vi "WS1050 36 DUT Reliability HD_Cycling Ver1.3.vi"() -> ()   [LabVIEW 2012]
uses:
  WS_VCAP Driver 029/Source/WSVCAP Shell/Type Defs/WSVCAP SHL I2C DUT Mask Mode Enum.ctl
  <vilib>/Utility/file.llb/Read From Spreadsheet File (DBL).vi
  All Driver/Keithley/2012_Keithley 24XX/Keithley 24XX.lvlib
panel:
  out "VISA resource name out":refnum<visa-resource-name>="GPIB0::3::INSTR"
  out "error out 2":errorcluster={"status"=TRUE, "code"=-63192, "source"="niLvFpga_Open_PXI-7813R.vi"}
  in  "Reg1_Bit Cntrl":string[](array[string])=["01", "02", "04", "08", "10", "20", "40", "80", "03", "06", "0C", "D8", "33", "66", "CC", "07", "0E", "1C", "38", "70", "E0", "0F", "1E", "3C", "78", "F0", "1F", "3E", "7C", "F8", "3F", "7E", "FC", "7F", "FE", "FD", "FB", "F7", "EF", "DF", "BF", "7F", "FC", "F9", "F3", "E7", "CF", "9F", "3F", "F8", "F1", "E3", "C7", "8F", "1F", "F0", "E1", "C3", "87", "0F", "E0", "C1", "83", "07", "C0", "81", "03", "AA", "55", "00"]
  out "date string":string="5/19/2014"
  out "PS1 Out":refnum<visa-resource-name>
  out "Ke2000 Out":refnum<visa-resource-name>="GPIB0::9::INSTR"
  in  "VPI_Cmd":string[](array[string])=["00", "3B", "00"]
  in  "VPI Name":string[](array[string])=["All_Drivers OFF", "All Drivers ON", "All Drivers OFF2"]
  in  "Tab Control":T1(tab)
  in  "No of Cmd":i64=3
  in  "Board#":string="BRD5"
  in  "Serial Number":string[][](table)=[["DUT", "SN"], ["DUT1", "1"], ["DUT2", "2"], ["DUT3", "3"], ["DUT4", "4"], ["DUT5", "5"], ["DUT6", "6"], ["DUT7", "7"], ["DUT8", "8"], ["DUT9", "9"], ["DUT10", "10"], ["DUT11", "11"], ["DUT12", "12"], ["DUT13", "13"], ["DUT14", "14"], ["DUT15", "15"], ["DUT16", "16"], ["DUT17", "17"], ["DUT18", "18"], ["DUT19", "19"], ["DUT20", "20"], ["DUT21", "21"], ["DUT22", "22"], ["DUT23", "23"], ["DUT24", "24"], ["DUT25", "25"], ["DUT26", "26"], ["DUT27", "27"], ["DUT28", "28"], ["DUT29", "29"], ["DUT30", "30"], ["DUT31", "31"], ["DUT32", "32"], ["DUT33", "33"], ["DUT34", "34"], ["DUT35", "35"], ["DUT36", "36"]]
  in  "SPI Clock Rate (Hz)":dbl=5000000.0 caption="Cycle Speed" format="%.1p Hz"
  in  "Wafer#":string="T7-EB"
  in  "File Name":string="CYC_WS1050_T7_EB_65C_40V_25DC_EMPTY_BRD5_141017_1"
  in  "TMN DC\\CAP Data Log File Path":path=path "C:/WS1050 36 DUT Data"
  in  "Test Program":string="WS1050 36 DUT Reliability HD_Cycling Ver1.3"
  out "Current Date":string="8/28/2014"
  out "Current Time":string="0950"
  in  "Start Date":string="10/21/2014"
  in  "Start Time":string="1542"
  in  "Comment":string="CYC65C40V"
  in  "OK Button":bool
  in  "Calibration":bool
  in  "Verify CP":bool
  in  "CP Setting":i32(ring) items=["CP OFF", "CP ON", "CP 35V", "CP 40V", "DVA ON", "DVA OFF", "REG1 ON", "REG1 OFF", "REG2 ON", "REG2 OFF", "REG3 ON", "REG3 OFF"]
  in  "Stop Calibration":bool
  in  "Set VDD":dbl=3.3 format="%.3g"
  in  "Command":string[](array[string])=["07020100003B", "070201003B00", "0702013B0000"]
  in  "Clock Rate (Hz)":dbl=1000000.0 caption="Meas Speed" format="%.1p Hz"
  out "AR  Measurent(Hz)":dbl
  in  "PS1 Source":refnum<visa-resource-name>="GPIB0::5::INSTR"
  in  "Ke2000":refnum<visa-resource-name>="GPIB0::9::INSTR"
  in  "CP to HD/Cycle":i32(ring)=1 items=["CP HDC 35V", "CP HDC 40.25V", "CP HDC 27.5V", "CP HDC 30.5V", "CP HDC 44V"]
  out "Simulate FPGA":bool
  out "Online":bool
  out "AR Cycling(Hz)":dbl=5000000.0
  in  "Ke2400":refnum<visa-resource-name>="GPIB0::3::INSTR"
  in  "Initialize AD7747":bool
  in  "DUT Mask Mode":T2=enum."All"
  in  "RFFE Slave Address":u8=7 caption="Slave Address" format="0x%02x"
  out "Activity Log":string="05/19/2014 -- 12:24:35.853::WSVCAP::APP::Application Started\n05/19/2014 -- 12:24:37.606::WSVCAP::WSVCAP SHL::WR I2C-REG:0x0A;MASK:0xFFFFFFFFFFFF;C1 DATA:22:22:22:22:22:22:22:22:22:22:22:22:22:22:22:22;C2 DATA:22:22:22:22:22:22:22:22:22:22:22:22:22:22:22:22;C3 DATA:22:22:22:22:22:22:22:22:22:22:22:22:22:22:22:22\r\n05/19/2014 -- 12:24:37.773::WSVCAP::WSVCAP SHL::WR I2C-ST:0,0,4,1\r\n05/19/2014 -- 12:24:37.903::WSVCAP::WSVCAP SHL::RD I2C-BYTES:4;ADD:0x00;MASK:0xFFFFFFFFFFFF\r\n05/19/2014 -- 12:24:38.045::WSVCAP::WSVCAP SHL::RD I2C:C1 DATA:2:2:2:2:2:2:2:2:2:2:2:2:2:2:2:2|A7:A9:AA:82:82:7F:82:81:82:81:83:82:81:82:82:81|46:36:BB:88:44:A3:E9:2B:32:20:ED:25:BB:3D:68:B|2C:6A:EB:A7:22:56:FE:CC:36:82:D7:B0:3B:48:F9:CC;C2 DATA:2:2:2:2:2:2:2:2:2:2:2:2:2:2:2:2|94:94:94:80:80:80:80:80:81:7E:7E:81:80:7E:80:80|47:33:15:82:62:B:E8:1C:D7:C3:7D:41:7C:B7:4C:2A|C4:B4:AE:8:1E:D1:4E:37:11:C0:6F:63:42:9D:63:B5;C3 DATA:2:2:2:2:2:2:2:2:2:2:2:2:2:2:2:2|95:95:95:81:81:7E:81:80:84:7D:80:83:81:7E:7F:80|AB:C4:14:B5:7B:52:DF:C9:79:5D:5F:30:99:31:1E:F4|6E:5C:F7:A8:C3:EB:7B:EF:33:92:89:77:4D:67:75:DD;STATUS:0:0:4:0\r\n05/19/2014 -- 12:24:38.046::WSVCAP::WSVCAP SHL::WR I2C-REG:0x0A;MASK:0xFFFFFFFFFFFF;C1 DATA:22:22:22:22:22:22:22:22:22:22:22:22:22:22:22:22;C2 DATA:22:22:22:22:22:22:22:22:22:22:22:22:22:22:22:22;C3 DATA:22:22:22:22:22:22:22:22:22:22:22:22:22:22:22:22\r\n05/19/2014 -- 12:24:38.089::WSVCAP::WSVCAP SHL::WR I2C-ST:0,0,4,1\r\n05/19/2014 -- 12:24:38.219::WSVCAP::WSVCAP SHL::RD I2C-BYTES:4;ADD:0x00;MASK:0xFFFFFFFFFFFF\r\n05/19/2014 -- 12:24:38.362::WSVCAP::WSVCAP SHL::RD I2C:C1 DATA:2:2:2:2:2:2:2:2:2:2:2:2:2:2:2:2|A7:AB:AA:82:82:82:83:83:82:82:82:82:7F:82:82:81|4B:32:96:83:3E:61:43:17:25:62:AB:4D:A2:40:2E:5|3C:76:2B:B4:EE:E4:A9:1A:AA:A:26:C7:21:2E:87:5B;C2 DATA:2:2:2:2:2:2:2:2:2:2:2:2:2:2:2:2|94:94:94:80:80:80:80:80:80:7F:80:81:80:80:7F:80|4A:32:19:7D:19:6C:79:46:61:7F:4B:B8:A5:30:F3:14|B4:70:A:8C:9C:DC:43:FA:1E:A:C6:21:A:A9:13:F3;C3 DATA:2:2:2:2:2:2:2:2:2:2:2:2:2:2:2:2|95:97:94:81:80:81:82:81:80:7E:81:84:7F:81:80:80|B2:32:D0:A7:9E:4C:AB:D4:EE:D9:F0:82:B7:91:7:FF|C1:91:B6:3D:D8:E:1B:4F:9F:6A:F1:6C:E7:3F:7:BA;STATUS:0:0:4:0\r\n05/19/2014 -- 12:24:38.364::WSVCAP::WSVCAP SHL::WR I2C-REG:0x0A;MASK:0xFFFFFFFFFFFF;C1 DATA:22:22:22:22:22:22:22:22:22:22:22:22:22:22:22:22;C2 DATA:22:22:22:22:22:22:22:22:22:22:22:22:22:22:22:22;C3 DATA:22:22:22:22:22:22:22:22:22:22:22:22:22:22:22:22\r\n05/19/2014 -- 12:24:38.406::WSVCAP::WSVCAP SHL::WR I2C-ST:0,0,4,1\r\n05/19/2014 -- 12:24:38.536::WSVCAP::WSVCAP SHL::RD I2C-BYTES:4;ADD:0x00;MASK:0xFFFFFFFFFFFF\r\n05/19/2014 -- 12:24:38.678::WSVCAP::WSVCAP SHL::RD I2C:C1 DATA:2:2:2:2:2:2:2:2:2:2:2:2:2:2:2:2|A7:A9:AB:82:82:81:82:82:82:82:82:82:82:82:82:81|46:71:4C:87:43:3D:7F:FC:25:4F:8E:54:97:3E:60:8C|AA:F4:1F:B5:CE:43:1F:36:9:87:9C:78:86:5:B6:8E;C2 DATA:2:2:2:2:2:2:2:2:2:2:2:2:2:2:2:2|94:94:94:80:7F:7F:80:80:80:80:80:81:80:80:80:80|49:36:18:7D:6E:C5:E4:3C:81:2E:41:D3:75:71:E3:72|E8:D3:E6:D1:E0:48:AE:D4:54:D:E8:8E:B4:41:68:4;C3 DATA:2:2:2:2:2:2:2:2:2:2:2:2:2:2:2:2|95:95:95:81:7F:7F:81:81:81:81:81:84:81:81:82:81|B3:F5:90:AB:82:69:7B:93:D0:77:E8:D5:E8:8C:84:E8|B9:AC:EE:2B:B6:71:8F:4A:74:31:56:BB:8A:B7:A0:C8;STATUS:0:0:4:0\r\n05/19/2014 -- 12:24:38.681::WSVCAP::WSVCAP SHL::WR I2C-REG:0x0A;MASK:0xFFFFFFFFFFFF;C1 DATA:22:22:22:22:22:22:22:22:22:22:22:22:22:22:22:22;C2 DATA:22:22:22:22:22:22:22:22:22:22:22:22:22:22:22:22;C3 DATA:22:22:22:22:22:22:22:22:22:22:22:22:22:22:22:22\r\n05/19/2014 -- 12:24:38.723::WSVCAP::WSVCAP SHL::WR I2C-ST:0,0,4,1\r\n05/19/2014 -- 12:24:38.854::WSVCAP::WSVCAP SHL::RD I2C-BYTES:4;ADD:0x00;MASK:0xFFFFFFFFFFFF\r\n05/19/2014 -- 12:24:38.996::WSVCAP::WSVCAP SHL::RD I2C:C1 DATA:2:2:2:2:2:2:2:2:2:2:2:2:2:2:2:2|A7:A9:AA:82:82:7F:83:81:82:81:84:82:7F:82:7F:82|43:FB:E:7F:3C:AD:35:35:26:A2:6C:21:4B:3D:8:6|63:9A:E1:F3:95:32:91:42:90:3C:78:1F:5C:D7:5F:D8;C2 DATA:2:2:2:2:2:2:2:2:2:2:2:2:2:2:2:2|94:94:94:80:80:80:80:80:81:80:7E:81:80:7E:7F:80|48:36:18:7F:5E:3D:69:83:DE:AE:A1:9E:31:AE:BB:96|15:A0:44:17:13:FD:CC:C8:6D:B2:EF:A7:C:C7:3B:F;C3 DATA:2:2:2:2:2:2:2:2:2:2:2:2:2:2:2:2|95:96:94:81:81:7E:82:80:84:80:80:84:7F:7E:7D:82|AD:3B:6D:A9:7C:57:9D:F5:7A:96:23:5C:36:2D:ED:5A|CD:46:DB:3B:C7:BD:70:60:33:B8:B:F7:63:A:51:4D;STATUS:0:0:4:0\r\n05/19/2014 -- 12:24:38.998::WSVCAP::WSVCAP SHL::WR I2C-REG:0x0A;MASK:0xFFFFFFFFFFFF;C1 DATA:22:22:22:22:22:22:22:22:22:22:22:22:22:22:22:22;C2 DATA:22:22:22:22:22:22:22:22:22:22:22:22:22:22:22:22;C3 DATA:22:22:22:22:22:22:22:22:22:22:22:22:22:22:22:22\r\n05/19/2014 -- 12:24:39.040::WSVCAP::WSVCAP SHL::WR I2C-ST:0,0,4,1\r\n05/19/2014 -- 12:24:39.170::WSVCAP::WSVCAP SHL::RD I2C-BYTES:4;ADD:0x00;MASK:0xFFFFFFFFFFFF\r\n05/19/2014 -- 12:24:39.311::WSVCAP::WSVCAP SHL::RD I2C:C1 DATA:2:2:2:2:2:2:2:2:2:2:2:2:2:2:2:2|A7:AA:AB:82:82:81:82:81:82:81:82:82:82:82:7F:82|44:F1:90:87:45:44:C8:2C:2C:F1:FC:1B:94:3B:3C:75|4A:49:95:19:99:73:64:3:23:24:F3:A2:5E:7F:C4:B6;C2 DATA:2:2:2:2:2:2:2:2:2:2:2:2:2:2:2:2|94:94:94:80:80:80:80:7F:80:80:7E:80:80:7E:7F:80|4C:36:17:7D:A8:9F:DE:C7:53:6D:8A:F4:41:A5:C6:E0|90:2E:24:C:D9:22:E4:76:3B:40:1D:53:33:B1:3E:4D;C3 DATA:2:2:2:2:2:2:2:2:2:2:2:2:2:2:2:2|95:97:95:81:81:7F:81:80:80:81:7F:82:81:7E:7D:82|AE:2B:A7:AB:CC:CD:A4:38:FD:17:80:F2:92:2D:45:C4|76:E5:D:B9:AD:B5:BA:8D:28:32:9E:42:B7:20:4A:D9;STATUS:0:0:4:0\r\n05/19/2014 -- 12:24:39.313::WSVCAP::WSVCAP SHL::WR I2C-REG:0x0A;MASK:0xFFFFFFFFFFFF;C1 DATA:22:22:22:22:22:22:22:22:22:22:22:22:22:22:22:22;C2 DATA:22:22:22:22:22:22:22:22:22:22:22:22:22:22:22:22;C3 DATA:22:22:22:22:22:22:22:22:22:22:22:22:22:22:22:22\r\n05/19/2014 -- 12:24:39.355::WSVCAP::WSVCAP SHL::WR I2C-ST:0,0,4,1\r\n05/19/2014 -- 12:24:39.486::WSVCAP::WSVCAP SHL::RD I2C-BYTES:4;ADD:0x00;MASK:0xFFFFFFFFFFFF\r\n05/19/2014 -- 12:24:39.628::WSVCAP::WSVCAP SHL::RD I2C:C1 DATA:2:2:2:2:2:2:2:2:2:2:2:2:2:2:2:2|A7:A9:AA:82:82:82:83:82:82:82:82:82:7F:82:7F:82|47:18:E4:87:3E:E7:6:65:25:92:37:38:A8:3E:89:85|7C:A7:7:2B:A3:7A:EC:EF:89:ED:F4:D3:D8:BC:3A:F5;C2 DATA:2:2:2:2:2:2:2:2:2:2:2:2:2:2:2:2|94:94:94:80:7F:80:80:7F:81:80:7E:80:80:80:81:80|49:37:17:80:76:25:6A:F8:DF:55:97:4D:B8:5B:2B:B1|13:E3:9A:3E:1A:2D:4F:B6:DB:E9:61:FA:8B:D6:9:CC;C3 DATA:2:2:2:2:2:2:2:2:2:2:2:2:2:2:2:2|95:95:95:81:7F:80:82:81:84:80:7F:81:80:81:7F:82|AF:93:3B:AF:5B:11:82:E4:7E:C3:2D:72:9:96:D9:A|DB:96:F2:10:5F:64:9A:C6:98:12:27:7D:10:D3:20:D9;STATUS:0:0:4:0\r\n05/19/2014 -- 12:24:40.132::WSVCAP::WSVCAP SHL::CLOSE\r\n"
  in  "C1 Cap DAC":u8=128 caption="B Data In" format="0x%02x"
  in  "C2 Cap DAC":u8=128 caption="B Data In" format="0x%02x"
  in  "C3 Cap DAC":u8=128 caption="B Data In" format="0x%02x"
  out "IDD Brd(uA)":string
  in  "CP to Meas":i32(ring)=1 items=["CP HDC 35V", "CP HDC 40.25V", "CP HDC 27.5V", "CP HDC 30.5V", "CP HDC 44V"]
  in  "CP VPI":i32(ring) items=["CP HDC 35V", "CP HDC 40.25V", "CP HDC 27.5V", "CP HDC 30.5V", "CP HDC 44V"]
  in  "Repeat Meas(s)":u32=900
  in  "Real No. From\nLookup Table":bool
  in  "Control Panel":T3={"Verify Socket"=FALSE, "HD/CYC"=FALSE, "E-CAL"=FALSE, "DVA"=FALSE, "VPI"=TRUE, "VSA"=TRUE, "HS"=TRUE}
  out "Verify Socket":bool
  out "HD/CYC":bool
  out "E-CAL":bool
  out "DVA":bool
  out "VPI":bool
  out "VSA":bool
  out "HS":bool
  in  "Lot#":string="WS1050"
  out "AD7747 Values":string[][](table)
  in  "Freq(Hz)":string="12K"
  in  "Reset P/S":bool
  in  "Test Sequences":i32(ring) items=["C1_C2_C3", "C2_C1_C3", "C3_C2_C1"]
  in  "WS1050/51":bool=TRUE
  in  "CP with DVA ON":i32(ring) items=["CP HDC 35V", "CP HDC 40.25V", "CP HDC 27.5V", "CP HDC 30.5V", "CP HDC 44V"]
  in  "% Duty Cycle":string="33"
  in  "Cmd To HD":string="0702013B3B3B"
  in  "Post CMd Delay":dbl[](array[numeric])=[1.8e-05, 1.8e-05, 1.8e-05] min=0.0 max=0.5 format="%#.0p s"
  in  "Cmin/Act":bool=TRUE
  out "40V_1":string[][](table)
  out "NOM IDD OFF(uA)":string
  out "40V_2":string[][](table)
  out "40V_3":string[][](table)
  out "Total Time":u64
  in  "Set HD/Cycle \nto Complete":u64=50000000000
  out "No of HD/Cycle\nCompleted":u64
  out "Cycle Count":u64 min=1 max=4 step=1
  out "Loop \ncompleted":i32=1
  out "Previous Time":string="12:20:26 PM"
  out "STATUS":string="Idle...."
  out "Total Delta C2(pF)":string[](array[string])
  out "Total Delta C1(pF)":string[](array[string])
  out "Total Delta C3(pF)":string[](array[string])
  out "RB Reg for HD":string[](array[string])
  out "RB Reg for HD/Cycle":string[](array[string])
  out "VPI C2":string[][](table)
  out "VPI C3":string[][](table)
  out "NOM IDD ON (uA)":string
  out "IDD_HD/CYC (uA)":string="164.601255E+0"
  in  "stop During HD/Cycles":bool
  in  "stop":bool
  out "IDD Stdby(uA)":string="2.606990E+0"
  out "VPI C1":string[][](table)
  out "VSA_V1":string[][](table)
  out "VSA_V2":string[][](table)
  out "VSA_V3":string[][](table)
  in  "VSA Voltage(V)":dbl[](array[numeric])=[-10.0, 0.0, 10.0]
  in  "DC_Temp":i32=65
  in  "HD/CYC Temp":i32=65
  in  "Time All ON (s)":u32=120
  in  "Time All OFF (s)":u32=120
  in  "HD_DC (Min)":u64=259200
  out "LPs Count":i32
  in  "X Repeat":i32=100
  out "No LPs to RP":i32
  out "Run Loops":i32=1
  out "TTCompleted":u64=2000
  in  "TTF Completed":u64=50000000000
  out "% Delta C_T0":string[][](array[string])
  out "% Delta C":string[][](array[string])
  out "EFuse RB T0":string[](array[string])
  out "Current EFuse Read back":string[](array[string])
  out "EFuse Readback Status":bool[](array[boolean])
  in  "DeltaC Target Setting(pF)":dbl=7.375
  out "error out":errorcluster
  in  "error in (no error)":errorcluster
  in  "HD RP":dbl=60.0
  in  "Cycle RP":dbl=10000.0
  out "Min Plot_1":dbl[][](graph) caption="(Y) Multi Plot 2"
  out "Min Plot_2":dbl[][](graph) caption="(Y) Multi Plot 2"
  out "Min Plot_3":dbl[][](graph) caption="(Y) Multi Plot 2"
  in  "Debug":bool
  in  "No of Rows\nFrom Spread Sheet":i32
  in  "Plot Delta Cmin":bool=TRUE
  in  "Plot":T4(ring)
  # "Company:  WiSpry Inc\n20 Fairbanks Ste 198 Irvine CA 92618\n\nAuthor:  Andy V Tran\nCreated:  03/19/2015\nLabVIEW 2012 Pro\nTest Program:  WS1050 36 DUT Reliability HD_Cycling ver1.3\nFPGA: WS_VCAP Driver 029"
  # "Note for HD Duty Cycle:\n1.  Set time to start HD_DC (Min), default is 259200 (6 months) \n2.  Set Time for Duty Cycle ON/OFF, default setting is 2 minutes\n3.  No of Loops to RP = 3600s/(Time ALL ON(s) + Time ALL + OFF(s))\n4.  Set X Repeat = no of runs, default is 100 runs\n5.  Set TTF Completed to stop the test.\n\nVer 1.3 updated:\n1.  Added stress sequences; CMin/ON-OFF repeat measurement\n2.  Fill \"na\" to preadsheet with no test"
  # "Minutes"
  # "X1000"
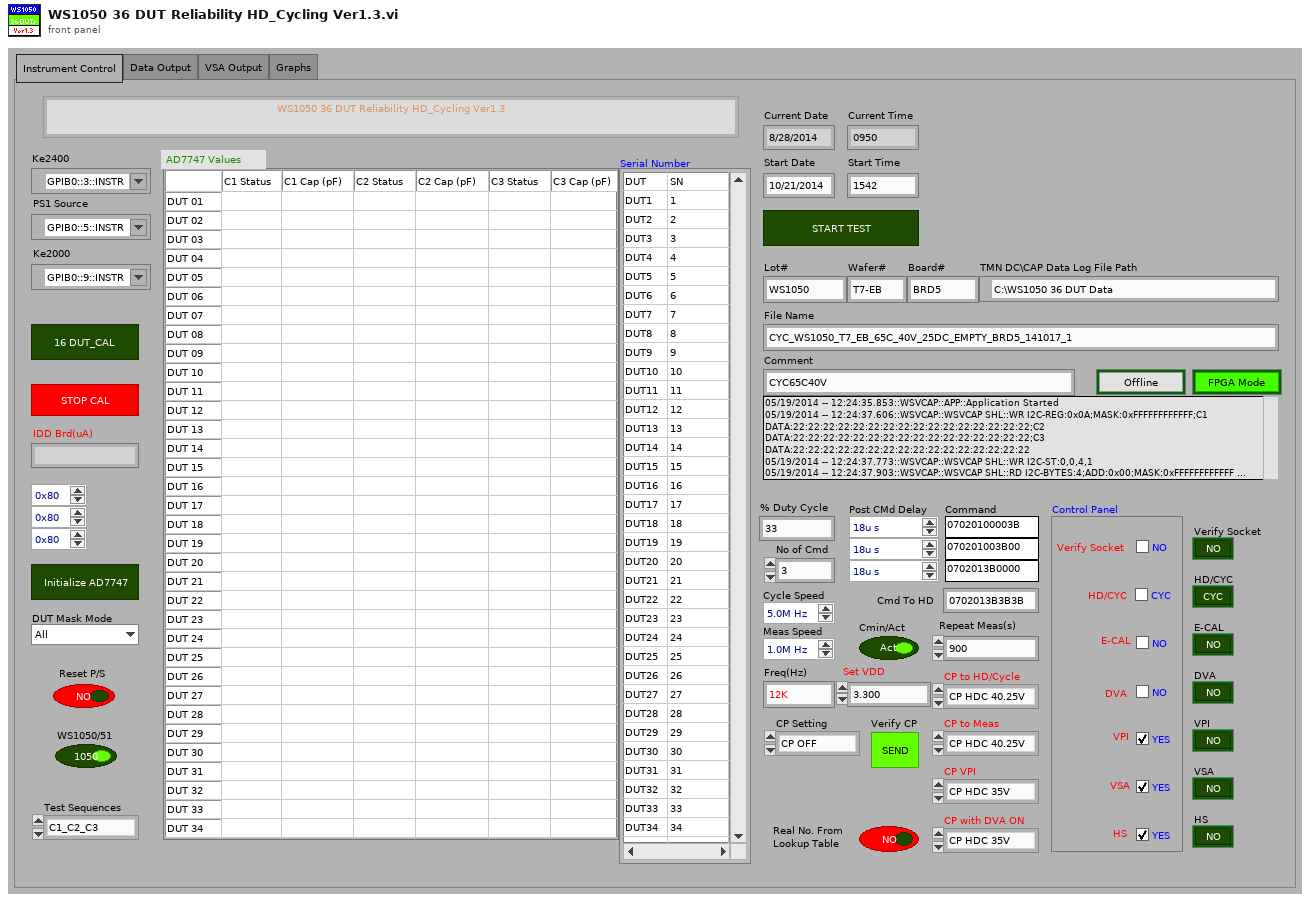
[diagram p1: front panel]
types:
  T1 = enum32{"Instrument Control", "Data Output", "VSA Output", "Graphs"}
  T2 = typedef "WSVCAP SHL I2C DUT Mask Mode Enum.ctl" = enum16{"Custom", "C1", "C2", "C3", "All"}
  T3 = cluster{"Verify Socket":bool, "HD/CYC":bool, "E-CAL":bool, "DVA":bool, "VPI":bool, "VSA":bool, "HS":bool}
  T4 = enum16{"ALL DUTs", "DUT 01", "DUT 02", "DUT 03", "DUT 04", "DUT 05", "DUT 06", "DUT 07", "DUT 08", "DUT 09", "DUT 10", "DUT 11", "DUT 12", "DUT 13", "DUT 14", "DUT 15", "DUT 16", "DUT 17", "DUT 18", "DUT 19", "DUT 20", "DUT 21", "DUT 22", "DUT 23", "DUT 24", "DUT 25", "DUT 26", "DUT 27", "DUT 28", "DUT 29", "DUT 30", "DUT 31", "DUT 32", "DUT 33", "DUT 34", "DUT 35", "DUT 36"}
  T5 = typedef "WSVCAP SHL Core System Cluster.ctl" = cluster{"Settings":T6, "FPGA Resource":tag, "Online":bool, "I2C Wait Ticks":u32, "SPI Wait Ticks":u32, "RFFE Wait Ticks":u32}
  T6 = typedef "WSVCAP SHL I2C Settings Cluster.ctl" = cluster{"FPGA Resource Name":string, "I2C Slave Address":u8, "I2C Clock Rate (Hz)":dbl, "SPI Clock Rate (Hz)":dbl, "RFFE Slave Address":u8, "RFFE Clock Rate (Hz)":dbl, "Simulate FPGA":bool, "C1 Cap DAC Default":u8, "C2 Cap DAC Default":u8, "C3 Cap DAC Default":u8}
  T7 = enum16{"Idle...", "Voltage 1", "Voltage 2", "Voltage 3"}[]
  T8 = cluster{"Test Program ":string, "Comment":string, "Data Out":string, "Data Out":string, "Data Out":string, string, "Data Out":string, "Data Out":string, "string":string, "Freq(Hz)":string, "Board#":string}
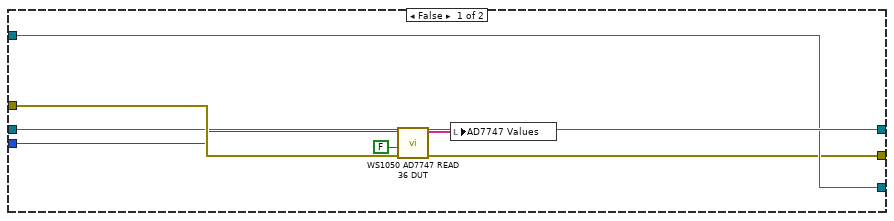
[diagram p10: hidden frame]
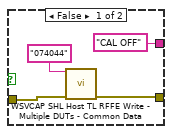
[diagram p11: hidden frame]
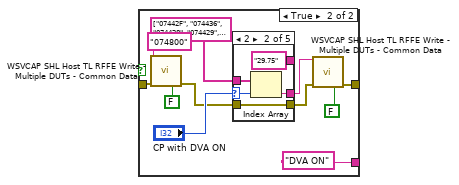
[diagram p12: hidden frame]
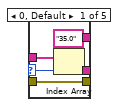
[diagram p13: hidden frame]
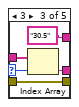
[diagram p14: hidden frame]
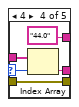
[diagram p15: hidden frame]
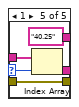
[diagram p16: hidden frame]
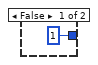
[diagram p17: hidden frame]
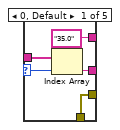
[diagram p18: hidden frame]
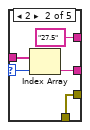
[diagram p19: hidden frame]
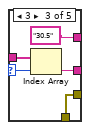
[diagram p20: hidden frame]
diagram:
  w19 = TRUE
  w25 = u16 0 items=["Off", "Moving Filter", "Repeating Filter"] ("Digital Filter (0: Off)")
  w26 = u16 7 items=["3.5 Digits"=4, "4.5 Digits"=5, "5.5 Digits"=6, "6.5 Digits"=7] ("Resolution (7: 6.5 digits)")
  n1 = case shown="True" w19 {
    tunnel: "error in (no error)" -> [w33 w34]
    tunnel: [w33 w41] -> w5
    frame False {
    }
    frame True {
      n2 = call "WSVCAP SHL Host TL Initialize.vi"("error in"=w34) -> ("error out"=w35:errorcluster)  [unwired: 13 in, 1 out]
      n3 = control-ref of="Activity Log"() -> (w37:refnum<vi>)
      n4 = call "ACT LG Activity Log Core.vi"("Display Ref"=w37, "Source"="WSVCAP", "Error In (no error)"=w35) -> ("Error Out"=w36:errorcluster)  [unwired: 11 in, 1 out]
      n5 = call "WSVCAP SHL Host TL Status Manager.vi"("error in"=w36) -> ("System Out"=w42:T5, "error out"=w41:errorcluster)  [unwired: 13 in]
      n6 = Unbundle By Name(w42) -> ("Online"=→"Online":bool, "Settings.Simulate FPGA"=→"Simulate FPGA":bool)
    }
  }
  n7 = case shown="True" TRUE {
    tunnel: w5 -> [w43 w48]
    tunnel: [w44 w47] -> w16
    tunnel: [w43 w46] -> w9
    tunnel: "Ke2400" -> [w44 w45]
    frame False {
    }
    frame True {
      n8 = VISA Write(VISA resource name=w45, write buffer="SOUR:FUNC VOLT;VOLT:MODE FIX;RANG 100;LEV 0.0;:SENS:FUNC \"CURR\";CURR:PROT 60E-3;RANG 100E-3;:OUTP ON", error in (no error)=w48) -> (VISA resource name out=w47:refnum<visa-resource-name>, error out=w46:errorcluster)  [unwired: 1 out]
    }
  }
  n9 = case shown="True" "Reset P/S" {
    tunnel: "PS1 Source" -> [w50 w57]
    tunnel: [w50 w55] -> w30
    tunnel: w5 -> [w51 w53]
    tunnel: [w51 w52] -> w4
    frame False {
    }
    frame True {
      n10 = call "Agilent 3631A Initialize.vi"("error in (no error)"=w53, "Default"=FALSE ("Reset? (T: Yes)"), "Reset"=TRUE ("ID Query? (T: Yes)"), "VISA resource name"=w57) -> ("error out"=w52:errorcluster, "VISA resource name out"=w55:refnum<visa-resource-name>)  [unwired: 6 in]
    }
  }
  n11 = call "Ke2000 Initialize.vi"("error in (no error)"=w5, "VISA resource name"="Ke2000") -> ("error out"=w27:errorcluster, "VISA resource name out"=w28:refnum<visa-resource-name>)  [unwired: 8 in]
  n12 = call "Ke2000 Configure DC Current.vi"("Resolution (7: 6.5 digits)"=w26, "Digital Filter (0: Off)"=w25, "Auto Range? (T: Auto)"=FALSE, "error in (no error)"=w27, "Custom Range (0 A)"=1.0, "VISA resource name"=w28) -> ("error out"=w6:errorcluster, "VISA resource name out"=w23:refnum<visa-resource-name>)  [unwired: 4 in]
  n13 = case shown="True" TRUE {
    tunnel: [_ w58] -> w32
    frame False {
    }
    frame True {
      n14 = call-poly <vilib>:"Read From Spreadsheet File.vi"("number of rows (all:-1)"=-1) -> ("all rows"=w58:dbl[][])  [unwired: 6 in, 4 out]
    }
  }
  n15 = Merge Errors(w9, w6, w4) -> (w17:errorcluster)
  n16 = while {
    tunnel: w17 -> [w62]
    tunnel: [w71] -> w13
    tunnel: w32 -> [w87]
    tunnel: w30 -> [w75]
    tunnel: w23 -> [w76]
    tunnel: [w85] -> w22
    tunnel: [w84] -> w21
    tunnel: w16 -> [w82]
    tunnel: [w81] -> w14
    tunnel: [FALSE ("stop")] -> w7
    i -> [w83]
    stop <- w88 stop-if-true
    n17 = case shown="0" w83 {
      tunnel: w62 -> [w99 w101]
      tunnel: [w98 w101] -> w78
      tunnel: "RFFE Slave Address" -> [w96 _]
      frame 0 {
        w92 = dbl[][] []
        w91 = "" ("uA")
        w93 = string[][] []
        w94 = string[] [] ("EFuse Read back")
        w100 = u64 0 ("No of HD/Cycle\nCompleted")
        n18 = local write "RB Reg for HD/Cycle"(w94) -> ()
        n19 = local write "Current EFuse Read back"(w94) -> ()
        n20 = local write "EFuse RB T0"(w94) -> ()
        n21 = local write "Total Delta C1(pF)"(w94) -> ()
        n22 = local write "Total Delta C2(pF)"(w94) -> ()
        n23 = local write "Total Delta C3(pF)"(w94) -> ()
        n24 = local write "No of HD/Cycle\nCompleted"(w100) -> ()
        n25 = local write "Cycle Count"(w100) -> ()
        n26 = local write "VPI C2"(w93) -> ()
        n27 = local write "VSA_V3"(w93) -> ()
        n28 = local write "VSA_V1"(w93) -> ()
        n29 = local write "40V_2"(w93) -> ()
        n30 = local write "40V_1"(w93) -> ()
        n31 = local write "NOM IDD OFF(uA)"(w91) -> ()
        n32 = local write "NOM IDD ON (uA)"(w91) -> ()
        n33 = local write "IDD Brd(uA)"(w91) -> ()
        n34 = local write "VSA_V2"(w93) -> ()
        n35 = local write "VPI C1"(w93) -> ()
        n36 = local write "VPI C3"(w93) -> ()
        n37 = local write "% Delta C"(w93) -> ()
        n38 = local write "% Delta C_T0"(w93) -> ()
        n39 = local write "40V_3"(w93) -> ()
        n40 = call "WSVCAP SHL Host TL RFFE Configure.vi"("RFFE Slave Address"=w96, "Clock Rate (Hz)"="Clock Rate (Hz)", "error in"=w99) -> ("Actual Rate (Hz)"=→"AR  Measurent(Hz)":dbl, "error out"=w98:errorcluster)  [unwired: 11 in]
        n41 = local write "Min Plot_3"(w92) -> ()
        n42 = local write "Min Plot_1"(w92) -> ()
        n43 = local write "Min Plot_2"(w92) -> ()
      }
      frame 1, Default {
      }
    }
    n44 = while {
      tunnel: ["stop"] -> w80
      tunnel: w78 -> [w127]
      tunnel: [w119] -> w72
      tunnel: w75 -> [w126]
      tunnel: w76 -> [w121]
      tunnel: [w122] -> w74
      tunnel: [w120] -> w73
      tunnel: [w117] -> w69
      tunnel: [w116] -> w68
      tunnel: [w115] -> w67
      tunnel: [w114] -> w66
      tunnel: [w113] -> w65
      tunnel: [w112] -> w64
      tunnel: [w111] -> w63
      tunnel: ["Command"] -> w61
      tunnel: ["Post CMd Delay"] -> w60
      stop <- w134 stop-if-true
      # "Set Date & Time to Start Test"
      n45 = case shown="True" "Initialize AD7747" {
        tunnel: w127 -> [w143 w148]
        tunnel: [w143 w144] -> w110
        tunnel: w126 -> [w142 w146]
        tunnel: [w142 w145] -> w125
        frame False {
        }
        frame True {
          w149 = T7 [enum."Voltage 2", enum."Voltage 3", enum."Voltage 1"] items=["Idle...", "Voltage 1", "Voltage 2", "Voltage 3"]
          n46 = for {
            tunnel: w146 -> [w159]
            tunnel: w149 -> [w157] mode=indexing
            tunnel: [w156] -> w145
            shift-right: [w152] -> w147
            shift-left: w148 -> [w160]
            n47 = local read "Set VDD"() -> (w155:dbl)
            n48 = call "E3631A_Voltage Controller.vi"("VISA resource name"=w159, "I_VDD(A)"=0.5, "Channel Controller"=w157, "Voltage 1"=w155, "Voltage 2"=3.3, "error in (no error)"=w160, "I_3.3V (A)"=0.5) -> ("VISA resource name out"=w156:refnum<visa-resource-name>, "error out"=w151:errorcluster)  [unwired: 7 in]
            n49 = call "Delay T4.vi"("milliseconds to wait"=u32 100, "error in (no error)"=w151) -> ("error out"=w152:errorcluster)  [unwired: 9 in]
          }
          n50 = call "WS1050_AD7747_Init 36DUT.vi"("error in"=w147) -> ("error out"=w144:errorcluster)  [unwired: 10 in]
        }
      }
      n51 = call "Time_stamp.vi"() -> ("date/time string"=w139:string, "date string"=w141:string)  [unwired: 2 in]
      "Current Date" <- w141
      "Current Time" <- w139
      n52 = Equal?(x=w141, y="Start Date") -> (x = y?=w137:bool)
      n53 = Equal?(x=w139, y="Start Time") -> (x = y?=w136:bool)
      n54 = And(x=w137, y=w136) -> (x .and. y?=w133:bool)
      n55 = Compound Arithmetic op=OR(w133, "OK Button", "stop") -> (w134:bool)
      n56 = case shown="True" "Calibration" {
        tunnel: w110 -> [w190 w207]
        tunnel: [w184 w204] -> w108
        tunnel: w125 -> [w189 w203]
        tunnel: "DUT Mask Mode" -> [w188 w199]
        tunnel: [w189 w198] -> w123
        tunnel: w121 -> [w187 w194]
        tunnel: [w187 w191] -> w120
        frame False {
          n57 = call "WS1050 AD7747 READ 36 DUT.vi"("error in"=w190, "Log (T)"=FALSE, "DUT Mask Mode (All)"=w188) -> ("error out"=w184:errorcluster, "AD7747 Values"=w185:string[][])  [unwired: 7 in]
          n58 = local write "AD7747 Values"(w185) -> ()
        }
        frame True {
          n59 = flat-sequence {
            tunnel: w207 -> [w216]
            tunnel: [w211] -> w206
            tunnel: w203 -> [w215]
            tunnel: [w214] -> w202
            tunnel: w199 -> [w213]
            tunnel: [w213] -> w200
            tunnel: w194 -> [w209]
            tunnel: [w208] -> w193
            tunnel: w206 -> [w240]
            tunnel: [w239] -> w205
            tunnel: w202 -> [w238]
            tunnel: [w238] -> w201
            tunnel: w200 -> [w237]
            tunnel: "C1 Cap DAC" -> [w233]
            tunnel: "C2 Cap DAC" -> [w232]
            tunnel: "C3 Cap DAC" -> [w231]
            tunnel: w193 -> [w230]
            tunnel: [w230] -> w192
            tunnel: w205 -> [w249]
            tunnel: [w252] -> w204
            tunnel: w201 -> [w251]
            tunnel: [w248] -> w198
            tunnel: w192 -> [w247]
            tunnel: [w247] -> w191
            frame #0 {
              w217 = T7 [enum."Voltage 2", enum."Voltage 3", enum."Voltage 1"] items=["Idle...", "Voltage 1", "Voltage 2", "Voltage 3"]
              n60 = for {
                tunnel: w215 -> [w228]
                tunnel: w217 -> [w226] mode=indexing
                tunnel: [w225] -> w214
                shift-right: [w223] -> w210
                shift-left: w216 -> [w229]
                n61 = local read "Set VDD"() -> (w220:dbl)
                n62 = call "E3631A_Voltage Controller.vi"("VISA resource name"=w228, "I_VDD(A)"=0.5, "Channel Controller"=w226, "Voltage 1"=w220, "Voltage 2"=3.3, "error in (no error)"=w229, "I_3.3V (A)"=0.5) -> ("VISA resource name out"=w225:refnum<visa-resource-name>, "error out"=w222:errorcluster)  [unwired: 7 in]
                n63 = call "Delay T4.vi"("milliseconds to wait"=u32 100, "error in (no error)"=w222) -> ("error out"=w223:errorcluster)  [unwired: 9 in]
              }
              n64 = call "Ke2000 Single Reading.vi"("error in (no error)"=w210, "VISA resource name"=w209) -> ("error out"=w211:errorcluster, "VISA resource name out"=w208:refnum<visa-resource-name>, "uA"=→"IDD Brd(uA)":string)  [unwired: 5 in, 2 out]
              n65 = One Button Dialog(message="Please verify all sockets should be empty...") -> ()  [unwired: 1 in, 1 out]
            }
            frame #1 {
              n66 = call "WS1050 CAPDAC Setting.vi"("DUT Mask Mode (All)"=w237, "error in"=w240, "C3 Cap DAC"=w231, "C2 Cap DAC"=w232, "C1 Cap DAC"=w233) -> ("error out"=w235:errorcluster)  [unwired: 5 in, 1 out]
              n67 = call "WS1050 OFFSET CAL.vi"("error in"=w235, "OFFSET CAL"=TRUE ("Read?")) -> ("error out"=w234:errorcluster)  [unwired: 8 in, 1 out]
              n68 = while {
                tunnel: w234 -> [w246]
                tunnel: [w245] -> w239
                tunnel: w237 -> [w243]
                stop <- "Stop Calibration" stop-if-true
                n69 = call "WS1050 AD7747 READ 36 DUT.vi"("error in"=w246, "Log (T)"=FALSE, "DUT Mask Mode (All)"=w243) -> ("error out"=w245:errorcluster, "AD7747 Values"=→"AD7747 Values":string[][])  [unwired: 7 in]
              }
            }
            frame #2 {
              w250 = T7 [enum."Voltage 2", enum."Voltage 3", enum."Voltage 1"] items=["Idle...", "Voltage 1", "Voltage 2", "Voltage 3"]
              n70 = for {
                tunnel: w251 -> [w264]
                tunnel: w250 -> [w261] mode=indexing
                tunnel: [w260] -> w248
                shift-right: [w256] -> w252
                shift-left: w249 -> [w262]
                n71 = call "E3631A_Voltage Controller.vi"("VISA resource name"=w264, "I_VDD(A)"=0.5, "Channel Controller"=w261, "Voltage 1"=0.0, "Voltage 2"=3.3, "error in (no error)"=w262, "I_3.3V (A)"=0.5) -> ("VISA resource name out"=w260:refnum<visa-resource-name>, "error out"=w255:errorcluster)  [unwired: 7 in]
                n72 = call "Delay T4.vi"("milliseconds to wait"=u32 100, "error in (no error)"=w255) -> ("error out"=w256:errorcluster)  [unwired: 9 in]
              }
              n73 = One Button Dialog(message="Calibration Completed....") -> ()  [unwired: 1 in, 1 out]
            }
          }
        }
      }
      n74 = call "Control Panel.vi"("error in (no error)"=w110, "Control Panel"="Control Panel") -> ("error out"=w107:errorcluster, "VPI"=w113:bool, "DVA"=w114:bool, "E-CAL"=w115:bool, "VSA"=w112:bool, "HD/CYC"=w116:bool, "HS"=w111:bool, "Verify Socket"=w117:bool)  [unwired: 2 in]
      "Verify Socket" <- w117
      "E-CAL" <- w115
      "VPI" <- w113
      "VSA" <- w112
      "HS" <- w111
      "HD/CYC" <- w116
      "DVA" <- w114
      n75 = Merge Errors(w107, w108) -> (w109:errorcluster)
      n76 = case shown="True" "Verify CP" {
        tunnel: [w161 w165] -> w119
        tunnel: w123 -> [w162 w168]
        tunnel: [w162 w166] -> w122
        tunnel: w109 -> [w161 w164]
        frame False {
        }
        frame True {
          w169 = T7 [enum."Voltage 2", enum."Voltage 3", enum."Voltage 1"] items=["Idle...", "Voltage 1", "Voltage 2", "Voltage 3"]
          # "Verify CP"
          n77 = for {
            tunnel: w168 -> [w182]
            tunnel: w169 -> [w180] mode=indexing
            shift-right: [w177] -> w167
            shift-left: w164 -> [w183]
            tunnel: [w175] -> w166
            n78 = local read "Set VDD"() -> (w179:dbl)
            n79 = call "E3631A_Voltage Controller.vi"("VISA resource name"=w182, "I_VDD(A)"=0.5, "Channel Controller"=w180, "Voltage 1"=w179, "Voltage 2"=3.3, "error in (no error)"=w183, "I_3.3V (A)"=0.5) -> ("VISA resource name out"=w175:refnum<visa-resource-name>, "error out"=w178:errorcluster)  [unwired: 7 in]
            n80 = call "Delay T4.vi"("milliseconds to wait"=u32 100, "error in (no error)"=w178) -> ("error out"=w177:errorcluster)  [unwired: 9 in]
          }
          n81 = Index Array(array=string[] ["074000", "074040", "07476F", "074776", "074800", "074820", "07413B", "074100", "07423B", "074200", "07433B", "074300"], index="CP Setting") -> (element=w170:string)
          n82 = call "WSVCAP SHL Host TL RFFE Write - Multiple DUTs - Common Data.vi"("Data Out"=w170, "error in"=w167, "Log (T)"=FALSE) -> ("error out"=w165:errorcluster)  [unwired: 12 in]
        }
      }
      n83 = Array Subset(array="Post CMd Delay", length="No of Cmd") -> (w105:dbl[])  [unwired: 1 in]
      n84 = Array Subset(array="Command", length="No of Cmd") -> (w106:string[])  [unwired: 1 in]
      n85 = property on="Post CMd Delay" class="Arr (strict)"("Number of Rows"="No of Cmd") -> ()  [unwired: 2 in, 2 out]
      n86 = local write "Command"(w106) -> ()
      n87 = local write "Post CMd Delay"(w105) -> ()
      n88 = property on="Command" class="Arr (strict)"("Number of Rows"="No of Cmd") -> ()  [unwired: 2 in, 2 out]
      n89 = Wait Until Next ms Multiple(millisecond multiple=u32 100) -> ()  [unwired: 1 out]
    }
    n90 = case shown="False" w80 {
      tunnel: w72 -> [w324 w1871]
      tunnel: [w309 w1871] -> w71
      tunnel: w87 -> [w325 _]
      tunnel: w74 -> [w323 w1869]
      tunnel: w73 -> [w315 w1870]
      tunnel: [w321 w1870] -> w85
      tunnel: [w319 w1869] -> w84
      tunnel: w82 -> [w312 w1868]
      tunnel: [w308 w1868] -> w81
      tunnel: "RFFE Slave Address" -> [w303 _]
      tunnel: [FALSE ("stop During HD/Cycles") FALSE ("stop During HD/Cycles")] -> w70
      tunnel: w69 -> [w278 _]
      tunnel: w68 -> [w277 _]
      tunnel: w67 -> [w276 _]
      tunnel: w66 -> [w275 _]
      tunnel: w65 -> [w274 _]
      tunnel: w64 -> [w273 _]
      tunnel: w63 -> [w272 _]
      tunnel: w61 -> [w266 _]
      tunnel: w60 -> [w265 _]
      frame False {
        w304 = u64 0 ("Total Completed")
        w283 = u32 100 ("milliseconds to wait")
        w320 = T7 [enum."Voltage 2", enum."Voltage 3", enum."Voltage 1"] items=["Idle...", "Voltage 1", "Voltage 2", "Voltage 3"]
        w322 = T7 [enum."Voltage 2", enum."Voltage 3", enum."Voltage 1"] items=["Idle...", "Voltage 1", "Voltage 2", "Voltage 3"]
        # "VSA"
        # "HS"
        # "HD/CYC"
        # "DVA"
        # "E-CAL"
        # "VPI"
        # "Verify Socket"
        n91 = for {
          tunnel: w324 -> [w1866]
          tunnel: w323 -> [w1865]
          tunnel: w322 -> [w1863] mode=indexing
          tunnel: [w1858] -> w317
          tunnel: [w1862] -> w307
          n92 = local read "Set VDD"() -> (w1861:dbl)
          n93 = call "E3631A_Voltage Controller.vi"("VISA resource name"=w1865, "I_VDD(A)"=0.5, "Channel Controller"=w1863, "Voltage 1"=w1861, "Voltage 2"=3.3, "error in (no error)"=w1866, "I_3.3V (A)"=0.5) -> ("VISA resource name out"=w1862:refnum<visa-resource-name>, "error out"=w1859:errorcluster)  [unwired: 7 in]
          n94 = call "Delay T4.vi"("milliseconds to wait"=u32 100, "error in (no error)"=w1859) -> ("error out"=w1858:errorcluster)  [unwired: 9 in]
        }
        n95 = local write "Total Time"(w304) -> ()
        n96 = local write "TTCompleted"(w304) -> ()
        n97 = call "WSVCAP SHL Host TL RFFE Write - Multiple DUTs - Common Data.vi"("Data Out"="074000", "error in"=w317, "Log (T)"=FALSE) -> ("error out"=w318:errorcluster)  [unwired: 12 in]
        n98 = local read "IDD Brd(uA)"() -> (w292:string)
        n99 = call "Delay T4.vi"("milliseconds to wait"=w283, "error in (no error)"=w318) -> ("error out"=w316:errorcluster)  [unwired: 9 in]
        n100 = call "Ke2000 Single Reading.vi"("error in (no error)"=w316, "VISA resource name"=w315) -> ("error out"=w293:errorcluster, "VISA resource name out"=w314:refnum<visa-resource-name>, "uA"=w295:string)  [unwired: 5 in, 2 out]
        n101 = call "Substration.vi"("error in (no error)"=w293, "Input2"=w292, "Input1"=w295) -> ("error out"=w268:errorcluster, "In1 - In2"=w294:string)  [unwired: 7 in]
        "IDD Stdby(uA)" <- w294
        n102 = case shown="True" w277 {
          tunnel: [1 ("X Repeat") w386] -> w306
          frame False {
          }
          frame True {
            n103 = local read "X Repeat"() -> (w386:i32)
          }
        }
        n104 = call "WSVCAP SHL Host TL RFFE Write - Multiple DUTs - Common Data.vi"("Data Out"="074040", "error in"=w268, "Log (T)"=FALSE) -> ("error out"=w267:errorcluster)  [unwired: 12 in]
        n105 = call "Delay T4.vi"("milliseconds to wait"=w283, "error in (no error)"=w267) -> ("error out"=w301:errorcluster)  [unwired: 9 in]
        n106 = case shown="False" w275 {
          tunnel: w301 -> [w348 w357]
          tunnel: [w347 w355] -> w299
          tunnel: ["DVA OFF" ("Data Out") "DVA ON" ("Data Out")] -> w300
          frame False {
            n107 = call "WSVCAP SHL Host TL RFFE Write - Multiple DUTs - Common Data.vi"("Data Out"="074820", "error in"=w348) -> ("error out"=w347:errorcluster)  [unwired: 13 in]
          }
          frame True {
            n108 = call "WSVCAP SHL Host TL RFFE Write - Multiple DUTs - Common Data.vi"("Data Out"="074800", "error in"=w357, "Log (T)"=FALSE) -> ("error out"=w353:errorcluster)  [unwired: 12 in]
            n109 = case shown="2" "CP with DVA ON" {
              selector: "CP with DVA ON" -> [w363 w368 w373 w378 w382]
              tunnel: string[] ["07442F", "074436", "074428", "074429", "07443B"] -> [w364 w369 w374 w379 w384]
              tunnel: [w362 w367 w372 w377 w383] -> w349
              tunnel: ["35.0" ("Data Out") "29.75" ("Data Out") "30.5" ("Data Out") "44.0" ("Data Out") "40.25" ("Data Out")] -> _
              tunnel: w353 -> [w360 w365 w370 w375 w380]
              tunnel: [w360 w365 w370 w375 w380] -> w352
              frame 0, Default {
                n110 = Index Array(array=w364, index=w363) -> (element=w362:string)
              }
              frame 2 {
                n111 = Index Array(array=w369, index=w368) -> (element=w367:string)
              }
              frame 3 {
                n112 = Index Array(array=w374, index=w373) -> (element=w372:string)
              }
              frame 4 {
                n113 = Index Array(array=w379, index=w378) -> (element=w377:string)
              }
              frame 1 {
                n114 = Index Array(array=w384, index=w382) -> (element=w383:string)
              }
            }
            n115 = call "WSVCAP SHL Host TL RFFE Write - Multiple DUTs - Common Data.vi"("Data Out"=w349, "error in"=w352, "Log (T)"=FALSE) -> ("error out"=w355:errorcluster)  [unwired: 12 in]
          }
        }
        n116 = for {
          N: 36 -> [_]
          tunnel: "Serial Number" -> [w330]
          tunnel: [w328] -> w280 mode=indexing
          i -> [w327]
          n117 = Increment(x=w327) -> (x+1=w326:i32)
          n118 = Index Array(array=w330, index (row)=w326, index (col)=1 ("disabled index (col)")) -> (element=w328:string)
        }
        n119 = Not(x=w272) -> (.not. x?=w279:bool)
        n120 = Number To Fractional String(number="Set VDD", precision (6)=i16 2) -> (F-format string=w297:string)  [unwired: 2 in]
        n121 = call "Delay T4.vi"("milliseconds to wait"=w283, "error in (no error)"=w299) -> ("error out"=w287:errorcluster)  [unwired: 9 in]
        n122 = case shown="True" w276 {
          tunnel: w287 -> [w334 w336]
          tunnel: [w331 w335] -> w286
          tunnel: ["CAL OFF" ("Data Out") "CAL ON" ("Data Out")] -> w288
          frame False {
            n123 = call "WSVCAP SHL Host TL RFFE Write - Multiple DUTs - Common Data.vi"("Data Out"="074044", "error in"=w334) -> ("error out"=w331:errorcluster)  [unwired: 13 in]
          }
          frame True {
            n124 = for {
              tunnel: string[] ["074900", "074920", "074900"] -> [w344] mode=indexing
              tunnel: w336 -> [w341]
              tunnel: [w340] -> w335
              n125 = call "WSVCAP SHL Host TL RFFE Write - Multiple DUTs - Common Data.vi"("Data Out"=w344, "error in"=w341, "Log (T)"=FALSE) -> ("error out"=w343:errorcluster)  [unwired: 12 in]
              n126 = call "Delay T4.vi"("milliseconds to wait"=u32 10, "error in (no error)"=w343) -> ("error out"=w340:errorcluster)  [unwired: 9 in]
            }
          }
        }
        n127 = for {
          N: w306 -> [_]
          tunnel: w325 -> [w424]
          tunnel: [w420] -> w321
          tunnel: w294 -> [w419]
          tunnel: w314 -> [w418]
          tunnel: "TMN DC\\CAP Data Log File Path" -> [w417]
          tunnel: w312 -> [w415]
          tunnel: [w414] -> w310
          tunnel: w307 -> [w389]
          shift-right: [w409] -> _
          shift-left: u64 0 -> [w411]
          tunnel: w277 -> [w408]
          tunnel: w303 -> [w403]
          tunnel: w303 -> [w402]
          tunnel: w300 -> [w401]
          tunnel: w297 -> [w400]
          tunnel: [w399] -> w291
          tunnel: w288 -> [w398]
          tunnel: w286 -> [w397]
          tunnel: w275 -> [w396]
          tunnel: w278 -> [w394]
          tunnel: w274 -> [w393]
          tunnel: w279 -> [w392]
          tunnel: w273 -> [w391]
          tunnel: w280 -> [w390]
          tunnel: [w389] -> w269
          tunnel: w266 -> [w388]
          tunnel: w265 -> [w387]
          i -> [w407]
          stop <- w395 stop-if-true
          n128 = while {
            tunnel: w424 -> [w645]
            tunnel: w417 -> [w656]
            tunnel: "Lot#" -> [w655]
            tunnel: "Wafer#" -> [w654]
            tunnel: w390 -> [w653]
            tunnel: "Test Program" -> [w652]
            tunnel: w390 -> [w651]
            tunnel: "Comment" -> [w650]
            tunnel: "Lot#" -> [w649]
            tunnel: "Wafer#" -> [w648]
            tunnel: w418 -> [w644]
            tunnel: [w647] -> w420
            tunnel: w419 -> [w643]
            tunnel: w415 -> [w640]
            tunnel: [w639] -> w414
            tunnel: [w547] -> w405
            tunnel: w407 -> [w585]
            tunnel: [w576] -> w409
            tunnel: w411 -> [w575]
            shift-right: [w574] -> _
            shift-left: u64 0 -> [w468]
            tunnel: [w573] -> w404
            tunnel: w408 -> [w571]
            tunnel: w403 -> [w546]
            tunnel: w402 -> [w544]
            tunnel: w401 -> [w492]
            tunnel: w400 -> [w490]
            tunnel: [w465] -> w399
            tunnel: w398 -> [w472]
            tunnel: w397 -> [w471]
            tunnel: w396 -> [w470]
            tunnel: w394 -> [w462]
            tunnel: w393 -> [w461]
            tunnel: w392 -> [w456]
            tunnel: w391 -> [w450]
            tunnel: w388 -> [w426]
            tunnel: w387 -> [w425]
            i -> [w572]
            stop <- w586 stop-if-true
            n129 = case shown="4" "CP to HD/Cycle" {
              selector: "CP to HD/Cycle" -> [w660 w665 w670 w675 w679]
              tunnel: string[] ["07476F", "074776", "074765", "074769", "07477B"] -> [w661 w666 w671 w676 w681]
              tunnel: [w659 w664 w669 w674 w680] -> w487
              tunnel: ["35.0" ("Data Out") "27.5" ("Data Out") "30.5" ("Data Out") "44.0" ("Data Out") "40.25" ("Data Out")] -> w486
              tunnel: [w657 w662 w667 w672 w677] -> w485
              tunnel: w471 -> [w657 w662 w667 w672 w677]
              frame 0, Default {
                n130 = Index Array(array=w661, index=w660) -> (element=w659:string)
              }
              frame 2 {
                n131 = Index Array(array=w666, index=w665) -> (element=w664:string)
              }
              frame 3 {
                n132 = Index Array(array=w671, index=w670) -> (element=w669:string)
              }
              frame 4 {
                n133 = Index Array(array=w676, index=w675) -> (element=w674:string)
              }
              frame 1 {
                n134 = Index Array(array=w681, index=w679) -> (element=w680:string)
              }
            }
            n135 = flat-sequence {
              tunnel: [w749] -> w638
              tunnel: [w744] -> w637
              tunnel: w645 -> [w747]
              tunnel: [w746] -> w636
              tunnel: w644 -> [w724]
              tunnel: w643 -> [w745]
              tunnel: [w745] -> w635
              tunnel: [w691] -> w634
              tunnel: [w688] -> w633
              tunnel: w485 -> [w737]
              tunnel: w585 -> [w742]
              tunnel: w572 -> [w716]
              tunnel: [w716] -> w582
              tunnel: w572 -> [w741]
              tunnel: w571 -> [w739]
              tunnel: [w738] -> w570
              tunnel: [w697] -> w565
              tunnel: [w696] -> w564
              tunnel: [w695] -> w563
              tunnel: [w701] -> w553
              tunnel: [w698] -> w552
              tunnel: w546 -> [w736]
              tunnel: [w736] -> w545
              tunnel: w544 -> [w735]
              tunnel: [w700] -> w531
              tunnel: [w699] -> w505
              tunnel: [w734] -> w493
              tunnel: w487 -> [w732]
              tunnel: [w718] -> w484
              tunnel: [w717] -> w476
              tunnel: w462 -> [w712]
              tunnel: w461 -> [w711]
              tunnel: [w711] -> w460
              tunnel: w456 -> [w710]
              tunnel: [w710] -> w455
              tunnel: w450 -> [w709]
              tunnel: [w709] -> w449
              tunnel: [w704] -> w444
              tunnel: ["Test Sequences"] -> w440
              tunnel: "Real No. From\nLookup Table" -> [w694]
              tunnel: ["WS1050/51"] -> w434
              tunnel: ["Cmin/Act"] -> w430
              tunnel: w426 -> [w683]
              tunnel: w425 -> [w682]
              tunnel: w638 -> [w1064]
              tunnel: [w1060] -> w543
              tunnel: w637 -> [w1063]
              tunnel: w636 -> [w1069]
              tunnel: [w1069] -> w542
              tunnel: w635 -> [w1068]
              tunnel: w634 -> [w1062]
              tunnel: w633 -> [w1061]
              tunnel: [w1051] -> w541
              tunnel: [w1068] -> w540
              tunnel: [w1062] -> w539
              tunnel: [w1061] -> w538
              tunnel: w582 -> [w1066]
              tunnel: [w1066] -> w537
              tunnel: w570 -> [w1065]
              tunnel: [w1065] -> w536
              tunnel: [w1063] -> w535
              tunnel: w565 -> [w1059]
              tunnel: w564 -> [w1044]
              tunnel: w563 -> [w1045]
              tunnel: [w1056] -> w534
              tunnel: w553 -> [w1058]
              tunnel: w552 -> [w1056]
              tunnel: [w1052] -> w533
              tunnel: w545 -> [w1057]
              tunnel: [w1042] -> w532
              tunnel: w531 -> [w1042]
              tunnel: [w1044] -> w530
              tunnel: w505 -> [w1043]
              tunnel: [w1043] -> w504
              tunnel: [w1045] -> w502
              tunnel: w493 -> [w1055]
              tunnel: [w1054] -> w477
              tunnel: w476 -> [w1054]
              tunnel: w460 -> [w1050]
              tunnel: [w1050] -> w459
              tunnel: w455 -> [w1049]
              tunnel: [w1049] -> w454
              tunnel: w449 -> [w1048]
              tunnel: [w1048] -> w448
              tunnel: w444 -> [w1047]
              tunnel: [w1046] -> w443
              tunnel: w440 -> [w1040]
              tunnel: [w1040] -> w439
              tunnel: w434 -> [w1039]
              tunnel: [w1039] -> w433
              tunnel: w430 -> [w1038]
              tunnel: [w1038] -> w429
              tunnel: w543 -> [w1183]
              tunnel: [w1182] -> w529
              tunnel: w542 -> [w1194]
              tunnel: [w1194] -> w526
              tunnel: w541 -> [w1174]
              tunnel: [w1174] -> w524
              tunnel: w540 -> [w1193]
              tunnel: [w1193] -> w522
              tunnel: w539 -> [w1192]
              tunnel: [w1192] -> w520
              tunnel: w538 -> [w1191]
              tunnel: [w1191] -> w518
              tunnel: w537 -> [w1190]
              tunnel: [w1190] -> w516
              tunnel: w536 -> [w1189]
              tunnel: [w1189] -> w514
              tunnel: w535 -> [w1188]
              tunnel: [w1188] -> w512
              tunnel: w534 -> [w1187]
              tunnel: [w1187] -> w510
              tunnel: [w1179] -> w508
              tunnel: w533 -> [w1178]
              tunnel: w532 -> [w1185]
              tunnel: w530 -> [w1184]
              tunnel: w504 -> [w1171]
              tunnel: [w1171] -> w503
              tunnel: w502 -> [w1173]
              tunnel: [w1173] -> w501
              tunnel: [w1180] -> w500
              tunnel: [w1181] -> w478
              tunnel: w477 -> [w1181]
              tunnel: w459 -> [w1177]
              tunnel: [w1177] -> w458
              tunnel: w454 -> [w1176]
              tunnel: [w1176] -> w453
              tunnel: w448 -> [w1175]
              tunnel: [w1175] -> w447
              tunnel: w443 -> [w1172]
              tunnel: w439 -> [w1169]
              tunnel: [w1172] -> w438
              tunnel: [w1169] -> w437
              tunnel: w433 -> [w1168]
              tunnel: [w1168] -> w432
              tunnel: w429 -> [w1167]
              tunnel: [w1167] -> w428
              tunnel: w529 -> [w1275]
              tunnel: [w1274] -> w528
              tunnel: [w1270] -> w527
              tunnel: w526 -> [w1287]
              tunnel: [w1287] -> w525
              tunnel: w524 -> [w1264]
              tunnel: [w1264] -> w523
              tunnel: w522 -> [w1286]
              tunnel: [w1286] -> w521
              tunnel: w520 -> [w1285]
              tunnel: [w1285] -> w519
              tunnel: w518 -> [w1284]
              tunnel: [w1284] -> w517
              tunnel: w516 -> [w1283]
              tunnel: [w1283] -> w515
              tunnel: w514 -> [w1282]
              tunnel: [w1282] -> w513
              tunnel: w512 -> [w1281]
              tunnel: [w1281] -> w511
              tunnel: w510 -> [w1280]
              tunnel: [w1280] -> w509
              tunnel: w508 -> [w1279]
              tunnel: [w1279] -> w507
              tunnel: [w1261] -> w506
              tunnel: w503 -> [w1277]
              tunnel: w501 -> [w1276]
              tunnel: w500 -> [w1269]
              tunnel: ["DeltaC Target Setting(pF)"] -> w491
              tunnel: [w1272] -> w479
              tunnel: w478 -> [w1272]
              tunnel: w470 -> [w1271]
              tunnel: [w1271] -> w469
              tunnel: w458 -> [w1268]
              tunnel: [w1268] -> w457
              tunnel: w453 -> [w1267]
              tunnel: [w1267] -> w452
              tunnel: w447 -> [w1266]
              tunnel: [w1266] -> w446
              tunnel: w438 -> [w1265]
              tunnel: w437 -> [w1262]
              tunnel: [w1261] -> w435
              tunnel: w432 -> [w1260]
              tunnel: [w1260] -> w431
              tunnel: w428 -> [w1259]
              tunnel: [w1259] -> w427
              tunnel: [w1405] -> w632
              tunnel: [w1371] -> w631
              tunnel: w528 -> [w1409]
              tunnel: w527 -> [w1385]
              tunnel: [w1394] -> w630
              tunnel: [w1385] -> w629
              tunnel: [w1408] -> w628
              tunnel: [w1407] -> w627
              tunnel: w525 -> [w1406]
              tunnel: [w1406] -> w626
              tunnel: w523 -> [w1394]
              tunnel: w521 -> [w1404]
              tunnel: [w1404] -> w625
              tunnel: w519 -> [w1400]
              tunnel: [w1400] -> w624
              tunnel: w517 -> [w1399]
              tunnel: [w1399] -> w623
              tunnel: w515 -> [w1395]
              tunnel: [w1395] -> w581
              tunnel: w513 -> [w1403]
              tunnel: [w1403] -> w569
              tunnel: w511 -> [w1402]
              tunnel: [w1401] -> w566
              tunnel: w509 -> [w1397]
              tunnel: w507 -> [w1393]
              tunnel: [w1398] -> w562
              tunnel: [w1396] -> w561
              tunnel: [w1393] -> w556
              tunnel: w506 -> [w1392]
              tunnel: [w1379] -> w551
              tunnel: [w1378] -> w550
              tunnel: [w1377] -> w549
              tunnel: w491 -> [w1391]
              tunnel: [w1376] -> w480
              tunnel: w479 -> [w1376]
              tunnel: [w1375] -> w475
              tunnel: w469 -> [w1374]
              tunnel: w457 -> [w1369]
              tunnel: w452 -> [w1368]
              tunnel: [w1368] -> w451
              tunnel: w446 -> [w1367]
              tunnel: [w1367] -> w445
              tunnel: w435 -> [w1364]
              tunnel: w431 -> [w1363]
              tunnel: w427 -> [w1352]
              tunnel: w632 -> [w1612]
              tunnel: [w1612] -> w622
              tunnel: [w1597] -> w621
              tunnel: [w1611] -> w620
              tunnel: w631 -> [w1610]
              tunnel: w630 -> [w1609]
              tunnel: w629 -> [w1608]
              tunnel: [w1609] -> w619
              tunnel: [w1608] -> w618
              tunnel: w628 -> [w1607]
              tunnel: [w1607] -> w617
              tunnel: w627 -> [w1606]
              tunnel: [w1606] -> w616
              tunnel: w626 -> [w1605]
              tunnel: [w1605] -> w615
              tunnel: w625 -> [w1604]
              tunnel: [w1604] -> w614
              tunnel: w624 -> [w1603]
              tunnel: [w1603] -> w613
              tunnel: w623 -> [w1602]
              tunnel: [w1602] -> w612
              tunnel: w640 -> [w1601]
              tunnel: [w1599] -> w611
              tunnel: [w1579] -> w610
              tunnel: [w1580] -> w609
              tunnel: [w1578] -> w608
              tunnel: w581 -> [w1595]
              tunnel: [w1595] -> w580
              tunnel: w569 -> [w1594]
              tunnel: [w1594] -> w568
              tunnel: w566 -> [w1611]
              tunnel: w562 -> [w1592]
              tunnel: w561 -> [w1593]
              tunnel: [w1593] -> w560
              tunnel: [w1592] -> w558
              tunnel: w556 -> [w1591]
              tunnel: [w1591] -> w555
              tunnel: w551 -> [w1577]
              tunnel: w550 -> [w1576]
              tunnel: w549 -> [w1575]
              tunnel: [w1572] -> w548
              tunnel: [w1577] -> w499
              tunnel: [w1576] -> w497
              tunnel: [w1575] -> w495
              tunnel: [w1574] -> w481
              tunnel: w480 -> [w1574]
              tunnel: w475 -> [w1573]
              tunnel: [w1573] -> w474
              tunnel: w451 -> [w1572]
              tunnel: w445 -> [w1571]
              tunnel: w622 -> [w1707]
              tunnel: [w1707] -> w607
              tunnel: w621 -> [w1731]
              tunnel: [w1730] -> w606
              tunnel: w656 -> [w1732]
              tunnel: w655 -> [w1729]
              tunnel: w654 -> [w1728]
              tunnel: w653 -> [w1727]
              tunnel: [w1726] -> w605
              tunnel: w620 -> [w1720]
              tunnel: [w1720] -> w604
              tunnel: w619 -> [w1725]
              tunnel: w618 -> [w1724]
              tunnel: [w1725] -> w603
              tunnel: [w1724] -> w602
              tunnel: [w1715] -> w601
              tunnel: w617 -> [w1723]
              tunnel: [w1723] -> w600
              tunnel: w616 -> [w1722]
              tunnel: [w1722] -> w599
              tunnel: w615 -> [w1719]
              tunnel: [w1721] -> w598
              tunnel: w468 -> [w1718]
              tunnel: [w1717] -> w597
              tunnel: [w1705] -> w596
              tunnel: w614 -> [w1716]
              tunnel: w613 -> [w1714]
              tunnel: w612 -> [w1713]
              tunnel: "File Name" -> [w1712]
              tunnel: w611 -> [w1711]
              tunnel: [w1711] -> w595
              tunnel: w610 -> [w1710]
              tunnel: [w1710] -> w594
              tunnel: [w1709] -> w593
              tunnel: w609 -> [w1709]
              tunnel: w608 -> [w1708]
              tunnel: [w1708] -> w592
              tunnel: [w1703] -> w583
              tunnel: w580 -> [w1704]
              tunnel: [w1704] -> w578
              tunnel: w575 -> [w1702]
              tunnel: w568 -> [w1701]
              tunnel: [w1701] -> w567
              tunnel: w560 -> [w1700]
              tunnel: [w1700] -> w559
              tunnel: w558 -> [w1699]
              tunnel: [w1699] -> w557
              tunnel: w555 -> [w1698]
              tunnel: [w1698] -> w554
              tunnel: w548 -> [w1697]
              tunnel: w499 -> [w1696]
              tunnel: [w1696] -> w498
              tunnel: w497 -> [w1695]
              tunnel: [w1695] -> w496
              tunnel: w495 -> [w1694]
              tunnel: [w1694] -> w494
              tunnel: w484 -> [w1693]
              tunnel: [w1693] -> w483
              tunnel: [w1692] -> w482
              tunnel: w481 -> [w1692]
              tunnel: w474 -> [w1691]
              tunnel: [w1691] -> w473
              tunnel: ["Freq(Hz)"] -> w442
              tunnel: ["Board#"] -> w441
              tunnel: w607 -> [w1804]
              tunnel: w606 -> [w1803]
              tunnel: w656 -> [w1766]
              tunnel: w652 -> [w1798]
              tunnel: w651 -> [w1801]
              tunnel: w650 -> [w1797]
              tunnel: w649 -> [w1800]
              tunnel: w648 -> [w1796]
              tunnel: w605 -> [w1799]
              tunnel: [w1804] -> w588
              tunnel: [w1802] -> w589
              tunnel: w604 -> [w1794]
              tunnel: [w1794] -> w590
              tunnel: w603 -> [w1793]
              tunnel: w602 -> [w1778]
              tunnel: w601 -> [w1792]
              tunnel: w600 -> [w1791]
              tunnel: w599 -> [w1780]
              tunnel: [w1788] -> w591
              tunnel: w598 -> [w1790]
              tunnel: w597 -> [w1789]
              tunnel: w596 -> [w1788]
              tunnel: "File Name" -> [w1759]
              tunnel: w595 -> [w1787]
              tunnel: [w1787] -> w587
              tunnel: w594 -> [w1786]
              tunnel: w593 -> [w1785]
              tunnel: w592 -> [w1784]
              tunnel: [w1783] -> w584
              tunnel: w583 -> [w1783]
              tunnel: [w1762] -> w579
              tunnel: w578 -> [w1762]
              tunnel: w567 -> [w1782]
              tunnel: w559 -> [w1781]
              tunnel: w557 -> [w1779]
              tunnel: w554 -> [w1777]
              tunnel: w498 -> [w1776]
              tunnel: w496 -> [w1775]
              tunnel: w494 -> [w1774]
              tunnel: w492 -> [w1773]
              tunnel: w472 -> [w1772]
              tunnel: w486 -> [w1771]
              tunnel: w490 -> [w1770]
              tunnel: w483 -> [w1769]
              tunnel: w482 -> [w1768]
              tunnel: w473 -> [w1767]
              tunnel: [w1764] -> w467
              tunnel: [w1755] -> w463
              tunnel: w442 -> [w1754]
              tunnel: w441 -> [w1752]
              tunnel: [w1825] -> w646
              tunnel: [w1826] -> w647
              tunnel: [w1827] -> w547
              tunnel: w591 -> [w1818]
              tunnel: w590 -> [w1826]
              tunnel: w589 -> [w1814]
              tunnel: w588 -> [w1827]
              tunnel: w587 -> [w1820]
              tunnel: [w1820] -> w639
              tunnel: [w1817] -> w576
              tunnel: w584 -> [w1817]
              tunnel: w579 -> [w1819]
              tunnel: [w1819] -> w577
              tunnel: [w1818] -> w574
              tunnel: [w1816] -> w573
              tunnel: [w1813] -> w464
              tunnel: w467 -> [w1812]
              tunnel: w463 -> [w1810]
              frame #0 {
                w705 = FALSE ("Log (T)")
                n136 = call "WSVCAP SHL Host TL RFFE Write - Multiple DUTs - Common Data.vi"("Data Out"=w732, "error in"=w737, "Log (T)"=FALSE) -> ("error out"=w714:errorcluster)  [unwired: 12 in]
                n137 = Index Array(array=w747, index (row)=w741, index (col)=0 ("disabled index (col)")) -> (element=w740:dbl)
                n138 = for {
                  tunnel: string[] ["0760", "0767", "0768"] -> [w796] mode=indexing
                  tunnel: [w792] -> w722 mode=indexing
                  tunnel: w714 -> [w790]
                  tunnel: [w789] -> w715
                  i -> [w795]
                  n139 = call "Delay T4.vi"("milliseconds to wait"=u32 10, "error in (no error)"=w790) -> ("error out"=w797:errorcluster)  [unwired: 9 in]
                  n140 = call "WSVCAP SHL Host TL RFFE Read - Multiple DUTs - Common Data.vi"("Data Out"=w796, "error in"=w797, "Log (T)"=FALSE) -> ("RFFE Data In"=w794:string[], "error out"=w789:errorcluster)  [unwired: 11 in]
                  n141 = Index Array(array=w794, index=w795) -> (element=w791:string)
                  n142 = String Subset(string=w791, offset (0)=0) -> (substring=w792:string)  [unwired: 1 in]
                }
                "RB Reg for HD/Cycle" <- w722
                n143 = local read "IDD Brd(uA)"() -> (w731:string)
                n144 = call "Delay T4.vi"("milliseconds to wait"=u32 100, "error in (no error)"=w715) -> ("error out"=w727:errorcluster)  [unwired: 9 in]
                n145 = call "Ke2000 Single Reading.vi"("error in (no error)"=w727, "VISA resource name"=w724) -> ("error out"=w729:errorcluster, "VISA resource name out"=w693:refnum<visa-resource-name>, "uA"=w730:string)  [unwired: 5 in, 2 out]
                n146 = call "Substration.vi"("error in (no error)"=w729, "Input2"=w731, "Input1"=w730) -> ("error out"=w726:errorcluster, "In1 - In2"=→"IDD_HD/CYC (uA)":string)  [unwired: 7 in]
                n147 = case shown="False" w739 {
                  tunnel: [w828 w933] -> w749
                  tunnel: [w829 w918] -> w708
                  tunnel: [w827 w934] -> w746
                  tunnel: w726 -> [w823 w922]
                  tunnel: w742 -> [_ w924]
                  tunnel: w740 -> [w820 w919]
                  tunnel: [w825 w920] -> w738
                  tunnel: w716 -> [w812 w916]
                  tunnel: w735 -> [w822 _]
                  tunnel: ["% Duty Cycle" "100" ("Data Out")] -> w718
                  tunnel: w712 -> [w810 _]
                  tunnel: w694 -> [w809 w911]
                  tunnel: w683 -> [w806 _]
                  tunnel: w682 -> [w805 _]
                  frame False {
                    # "Cycles in 1s"
                    n148 = case shown="True" w809 {
                      tunnel: w823 -> [w835 w841]
                      tunnel: w820 -> [w834 w840]
                      tunnel: [w833 w841] -> w819
                      tunnel: w812 -> [w832 _]
                      tunnel: [w831 w840] -> w818
                      tunnel: [u64 1000 ("y") u64 1 ("y")] -> w813
                      frame False {
                        n149 = case shown="8, Default" w832 {
                          tunnel: w834 -> [w837 _]
                          tunnel: [w837 "Cycle RP"] -> w831
                          tunnel: [w836 w838] -> w833
                          tunnel: w835 -> [w836 w838]
                          frame 0..7 {
                          }
                          frame 8, Default {
                          }
                        }
                      }
                      frame True {
                        # "Read real number\nfrom lookup table"
                      }
                    }
                    n150 = call "WSVCAP SHL Host TL RFFE Configure.vi"("RFFE Slave Address"=w822, "Clock Rate (Hz)"="SPI Clock Rate (Hz)", "error in"=w819) -> ("Actual Rate (Hz)"=→"AR Cycling(Hz)":dbl, "error out"=w808:errorcluster)  [unwired: 11 in]
                    n151 = Array Max & Min(array=w805) -> (max value=w816:dbl)  [unwired: 3 out]
                    n152 = Divide(x=1.0, y=w816) -> (x/y=w815:dbl)
                    n153 = To Unsigned Quad Integer(1:w815) -> (0:w814:u64)
                    n154 = Not(x=w810) -> (.not. x?=w811:bool)
                    n155 = case shown="True" w811 {
                      tunnel: [w844 w866] -> w829
                      tunnel: [w847 w865] -> w828
                      tunnel: [u64 1 w864] -> w827
                      tunnel: w808 -> [w845 w863]
                      tunnel: w818 -> [_ w862]
                      tunnel: w805 -> [_ w860]
                      tunnel: w814 -> [_ w859]
                      tunnel: w813 -> [_ w858]
                      tunnel: w812 -> [w843 _]
                      tunnel: w806 -> [_ w857]
                      frame False {
                        n156 = case shown="1, Default" w843 {
                          tunnel: w845 -> [w848 w850]
                          tunnel: [w848 w849] -> w844
                          frame 0 {
                          }
                          frame 1, Default {
                            n157 = flat-sequence {
                              tunnel: "Repeat Meas(s)" -> [w856]
                              tunnel: w850 -> [w853]
                              tunnel: [w853] -> w849
                              frame #0 {
                                n158 = Multiply(x=w856, y=u32 1000) -> (x*y=w855:u32)
                                n159 = Wait (ms)(milliseconds to wait=w855) -> ()  [unwired: 1 out]
                                n160 = local write "STATUS"("Verify Sockets waiting times..." ("STATUS")) -> ()
                              }
                            }
                          }
                        }
                        n161 = local read "stop During HD/Cycles"() -> (w847:bool)
                      }
                      frame True {
                        n162 = while {
                          tunnel: w862 -> [w886]
                          tunnel: [w873] -> w866
                          tunnel: [w878] -> w865
                          tunnel: w863 -> [w884]
                          tunnel: [w872] -> w864
                          tunnel: w857 -> [w883]
                          tunnel: w860 -> [w882]
                          tunnel: w859 -> [w869]
                          tunnel: w858 -> [w867]
                          i -> [w881]
                          stop <- w877 stop-if-true
                          # "At least 1 second before target"
                          # "Remaining Cycles"
                          # "Target Cycles"
                          # "Cycles in 1s"
                          n163 = To Unsigned Quad Integer(1:w886) -> (0:w885:u64)
                          n164 = case shown="0" w881 {
                            tunnel: [w894 w896] -> w875
                            tunnel: w884 -> [w895 w896]
                            tunnel: w883 -> [w893 _]
                            tunnel: w882 -> [w892 _]
                            frame 0 {
                              n165 = call "WSVCAP SHL Host TL RFFE Write Cycle - Multiple DUTs - Common Data.vi"("Data Out (Cycle Commands)"=w893, "Post Command Delay"=w892, "error in"=w895, "Log (T)"=FALSE) -> ("error out"=w894:errorcluster)  [unwired: 11 in]
                            }
                            frame 1, Default {
                            }
                          }
                          n166 = Multiply(x=w885, y=w867) -> (x*y=w872:u64)
                          n167 = call "WSVCAP SHL Host TL SPI_RFFE Query Cycle Count.vi"("error in"=w875) -> ("Cycle Count"=w871:u64, "error out"=w880:errorcluster)  [unwired: 13 in]
                          "Cycle Count" <- w871
                          n168 = Subtract(x=w872, y=w871) -> (x-y=w870:u64)
                          n169 = Greater Or Equal?(x=w871, y=w872) -> (x >= y?=w879:bool)
                          n170 = local read "stop During HD/Cycles"() -> (w878:bool)
                          n171 = Greater?(x=w870, y=w869) -> (0:w868:bool)
                          n172 = case shown="True" w879 {
                            tunnel: [w898 w901] -> w874
                            tunnel: w880 -> [w898 w900]
                            tunnel: [FALSE TRUE] -> w876
                            frame False {
                            }
                            frame True {
                              n173 = call "WSVCAP SHL Host TL SPI Stop Write Cycle.vi"("error in"=w900) -> ("error out"=w901:errorcluster)  [unwired: 14 in]
                            }
                          }
                          n174 = Or(x=w876, y=w878) -> (x .or. y?=w877:bool)
                          n175 = case shown="True" w868 {
                            tunnel: w874 -> [w887 w890]
                            tunnel: [w887 w889] -> w873
                            frame False {
                            }
                            frame True {
                              n176 = call "MISC Wait with Data Flow.vi"("Error In (no error)"=w890, "Wait Time (500ms)"=u32 50) -> ("Error Out"=w889:errorcluster)  [unwired: 7 in, 2 out]
                            }
                          }
                        }
                        n177 = local write "STATUS"("Parts are Cycling...." ("STATUS")) -> ()
                      }
                    }
                    n178 = local read "HD/CYC Temp"() -> (w824:i32)
                    n179 = Number To Engineering String(4:w824) -> (0:w825:string)  [unwired: 3 in]
                  }
                  frame True {
                    n180 = case shown="False" w911 {
                      tunnel: w924 -> [w951 _]
                      tunnel: [w950 w963] -> w923
                      tunnel: w922 -> [w949 w964]
                      tunnel: [w948 w964] -> w921
                      tunnel: w919 -> [w947 w963]
                      tunnel: w916 -> [w946 _]
                      frame False {
                        n181 = case shown="1, Default" w951 {
                          tunnel: [w954 w961] -> w950
                          tunnel: w949 -> [w956 w962]
                          tunnel: [w955 w962] -> w948
                          tunnel: w947 -> [w953 _]
                          tunnel: w946 -> [w952 _]
                          frame 0 {
                            n182 = case shown="15, Default" w952 {
                              tunnel: [w957 "HD RP"] -> w954
                              tunnel: w956 -> [w958 w959]
                              tunnel: [w958 w959] -> w955
                              tunnel: w953 -> [w957 _]
                              frame 0..14 {
                              }
                              frame 15, Default {
                              }
                            }
                          }
                          frame 1, Default {
                            n183 = local read "HD RP"() -> (w961:dbl)
                          }
                        }
                      }
                      frame True {
                      }
                    }
                    n184 = call "WSVCAP SHL Host TL RFFE Write - Multiple DUTs - Common Data.vi"("Data Out"="Cmd To HD", "error in"=w921, "Log (T)"=FALSE) -> ("error out"=w907:errorcluster)  [unwired: 12 in]
                    n185 = local read "No of HD/Cycle\nCompleted"() -> (w925:u64)
                    n186 = call "Delay T4.vi"("milliseconds to wait"=u32 50, "error in (no error)"=w907) -> ("error out"=w904:errorcluster)  [unwired: 9 in]
                    n187 = for {
                      tunnel: string[] ["0761", "0762", "0763"] -> [w945] mode=indexing
                      tunnel: [w941] -> w903 mode=indexing
                      shift-right: [w938] -> w929
                      shift-left: w904 -> [w944]
                      i -> [w943]
                      n188 = call "WSVCAP SHL Host TL RFFE Read - Multiple DUTs - Common Data.vi"("Data Out"=w945, "error in"=w944, "Log (T)"=FALSE) -> ("RFFE Data In"=w940:string[], "error out"=w937:errorcluster)  [unwired: 11 in]
                      n189 = Index Array(array=w940, index=w943) -> (element=w939:string)
                      n190 = call "Delay T4.vi"("milliseconds to wait"=u32 10, "error in (no error)"=w937) -> ("error out"=w938:errorcluster)  [unwired: 9 in]
                      n191 = String Subset(string=w939, offset (0)=0) -> (substring=w941:string)  [unwired: 1 in]
                    }
                    "RB Reg for HD" <- w903
                    n192 = Greater?(x="HD_DC (Min)", y=w925) -> (0:w926:bool)
                    n193 = case shown="True" w926 {
                      tunnel: [_ w975] -> w931
                      tunnel: [w966 w974] -> w930
                      tunnel: w929 -> [w966 w973]
                      tunnel: w923 -> [w965 w972]
                      tunnel: [w965 w972] -> w928
                      frame False {
                      }
                      frame True {
                        n194 = Multiply(x=1000.0, y=w972) -> (x*y=w970:dbl)
                        n195 = Multiply(x=60.0, y=w970) -> (x*y=w968:dbl)
                        n196 = local write "STATUS"("Parts are Holding Down..." ("STATUS")) -> ()
                        n197 = event shown="[0] Timeout" {
                          selector: _ -> [_ _]
                          dyn-events: _ -> [_ _]
                          timeout: w968 -> [_ _]
                          tunnel: ["stop During HD/Cycles" TRUE ("stop During HD/Cycles")] -> w975
                          tunnel: w973 -> [w976 w978]
                          tunnel: [w976 w978] -> w974
                          event Timeout {
                            n198 = event-data() -> ()  [unwired: 1 in, 2 out]
                          }
                          event "stop During HD/Cycles": Value Change {
                            n199 = event-data() -> ()  [unwired: 1 in, 2 out]
                          }
                        }
                      }
                    }
                    n200 = Greater Or Equal?(x=w925, y="HD_DC (Min)") -> (x >= y?=w932:bool)
                    n201 = To Unsigned Quad Integer(1:w923) -> (0:w934:u64)
                    n202 = Add(x="Time All OFF (s)", y="Time All ON (s)") -> (x+y=w913:u32)
                    n203 = To Double Precision Float(number=w913) -> (double precision float=w912:dbl)
                    n204 = Divide(x=w912, y=60.0) -> (x/y=w914:dbl)
                    n205 = case shown="False" w932 {
                      tunnel: [w982 w998] -> w933
                      tunnel: [w983 w990] -> w918
                      tunnel: w930 -> [w983 w997]
                      tunnel: w931 -> [w982 w996]
                      tunnel: w928 -> [_ w995]
                      tunnel: [w981 w993] -> w920
                      tunnel: w914 -> [_ w987]
                      tunnel: "Time All OFF (s)" -> [_ w985]
                      tunnel: "Time All ON (s)" -> [_ w984]
                      frame False {
                        n206 = Number To Engineering String(4:"HD/CYC Temp") -> (0:w981:string)  [unwired: 3 in]
                      }
                      frame True {
                        n207 = Divide(x=w995, y=w987) -> (x/y=w994:dbl)
                        n208 = call "WSVCAP SHL Host TL RFFE Write - Multiple DUTs - Common Data.vi"("Data Out"="070201000000", "error in"=w997, "Log (T)"=FALSE) -> ("error out"=w1000:errorcluster)  [unwired: 12 in]
                        n209 = Round To Nearest(number=w994) -> (nearest integer value=w989:dbl)
                        n210 = call "Delay T4.vi"("milliseconds to wait"=u32 50, "error in (no error)"=w1000) -> ("error out"=w991:errorcluster)  [unwired: 9 in]
                        n211 = To Long Integer(number=w989) -> (32bit integer=w988:i32)
                        "No LPs to RP" <- w988
                        n212 = for {
                          N: w988 -> [_]
                          tunnel: w996 -> [w1018]
                          tunnel: [w1017] -> w998
                          tunnel: w991 -> [w1007]
                          tunnel: [w1006] -> w990
                          tunnel: w985 -> [w1004]
                          tunnel: w984 -> [w1002]
                          i -> [w1016]
                          stop <- w1017 stop-if-true
                          w1005 = FALSE ("Log (T)")
                          w1003 = u32 1 ("milliseconds to wait")
                          n213 = Increment(x=w1016) -> (x+1=→"LPs Count":i32)
                          n214 = call "WSVCAP SHL Host TL RFFE Write - Multiple DUTs - Common Data.vi"("Data Out"="074776", "error in"=w1007, "Log (T)"=w1005) -> ("error out"=w1024:errorcluster)  [unwired: 12 in]
                          n215 = call "Delay T4.vi"("milliseconds to wait"=w1003, "error in (no error)"=w1024) -> ("error out"=w1023:errorcluster)  [unwired: 9 in]
                          n216 = local read "CP to HD/Cycle"() -> (w1009:i32)
                          n217 = call "WSVCAP SHL Host TL RFFE Write - Multiple DUTs - Common Data.vi"("Data Out"="070201000000", "error in"=w1010) -> ("error out"=w1020:errorcluster)  [unwired: 13 in]
                          n218 = call "WSVCAP SHL Host TL RFFE Write - Multiple DUTs - Common Data.vi"("Data Out"="0702013B3B3B", "error in"=w1023, "Log (T)"=w1005) -> ("error out"=w1013:errorcluster)  [unwired: 12 in]
                          n219 = call "Delay T4.vi"("milliseconds to wait"=w1003, "error in (no error)"=w1013) -> ("error out"=w1012:errorcluster)  [unwired: 9 in]
                          n220 = flat-sequence {
                            tunnel: w1020 -> [w1031]
                            tunnel: [w1029] -> w1006
                            tunnel: w1004 -> [w1026]
                            frame #0 {
                              n221 = local write "STATUS"("Now HD OFF Time..." ("STATUS")) -> ()
                              n222 = Multiply(x=w1026, y=u32 1000) -> (x*y=w1028:u32)
                              n223 = call "Delay T4.vi"("milliseconds to wait"=w1028, "error in (no error)"=w1031) -> ("error out"=w1029:errorcluster)  [unwired: 9 in]
                            }
                          }
                          n224 = Index Array(array=string[] ["07476F", "074776", "074765", "074769", "07477B"], index=w1009) -> (element=w1014:string)
                          n225 = call "WSVCAP SHL Host TL RFFE Write - Multiple DUTs - Common Data.vi"("Data Out"=w1014, "error in"=w1012, "Log (T)"=w1005) -> ("error out"=w1011:errorcluster)  [unwired: 12 in]
                          n226 = flat-sequence {
                            tunnel: [w1036] -> w1010
                            tunnel: w1011 -> [w1033]
                            tunnel: w1002 -> [w1032]
                            frame #0 {
                              n227 = local write "STATUS"("Now HD ON Time..." ("STATUS")) -> ()
                              n228 = Multiply(x=w1032, y=u32 1000) -> (x*y=w1035:u32)
                              n229 = call "Delay T4.vi"("milliseconds to wait"=w1035, "error in (no error)"=w1033) -> ("error out"=w1036:errorcluster)  [unwired: 9 in]
                            }
                          }
                          n230 = Unbundle By Name(w1006) -> ("status"=w1019:bool)
                          n231 = Or(x=w1019, y=w1018) -> (x .or. y?=w1017:bool)
                        }
                        n232 = Number To Engineering String(4:"DC_Temp") -> (0:w993:string)  [unwired: 3 in]
                      }
                    }
                  }
                }
                n233 = case shown="0, Default" "CP to Meas" {
                  selector: "CP to Meas" -> [w766 w771 w776 w781 w785]
                  tunnel: string[] ["07476F", "074776", "074765", "074769", "07477B"] -> [w767 w772 w777 w782 w787]
                  tunnel: [w765 w770 w775 w780 w786] -> w720
                  tunnel: [w764 w769 w774 w779 w784] -> w713
                  tunnel: w708 -> [w764 w769 w774 w779 w784]
                  tunnel: ["35.0" ("Data Out") "27.5" ("Data Out") "30.5" ("Data Out") "44.0" ("Data Out") "40.25" ("Data Out")] -> w717
                  frame 0, Default {
                    n234 = Index Array(array=w767, index=w766) -> (element=w765:string)
                  }
                  frame 2 {
                    n235 = Index Array(array=w772, index=w771) -> (element=w770:string)
                  }
                  frame 3 {
                    n236 = Index Array(array=w777, index=w776) -> (element=w775:string)
                  }
                  frame 4 {
                    n237 = Index Array(array=w782, index=w781) -> (element=w780:string)
                  }
                  frame 1 {
                    n238 = Index Array(array=w787, index=w785) -> (element=w786:string)
                  }
                }
                n239 = call "WSVCAP SHL Host TL RFFE Write - Multiple DUTs - Common Data.vi"("Data Out"=w720, "error in"=w713, "Log (T)"=w705) -> ("error out"=w733:errorcluster)  [unwired: 12 in]
                n240 = flat-sequence {
                  tunnel: w707 -> [w799]
                  tunnel: [w799] -> w703
                  frame #0 {
                    w801 = "0" ("NOM IDD OFF(uA)")
                    w802 = string[] []
                    w803 = string[][] []
                    n241 = To Long Integer(number=0.0 ("No of Loops to RP")) -> (32bit integer=w800:i32)
                    n242 = local write "NOM IDD ON (uA)"(w801) -> ()
                    n243 = local write "NOM IDD OFF(uA)"(w801) -> ()
                    n244 = local write "LPs Count"(w800) -> ()
                    n245 = local write "No LPs to RP"(w800) -> ()
                    n246 = local write "Total Delta C1(pF)"(w802) -> ()
                    n247 = local write "Total Delta C2(pF)"(w802) -> ()
                    n248 = local write "Total Delta C3(pF)"(w802) -> ()
                    n249 = local write "Current EFuse Read back"(w802) -> ()
                    n250 = local write "RB Reg for HD"(w802) -> ()
                    n251 = local write "RB Reg for HD/Cycle"(w802) -> ()
                    n252 = local write "VSA_V3"(w803) -> ()
                    n253 = local write "VSA_V1"(w803) -> ()
                    n254 = local write "VSA_V2"(w803) -> ()
                    n255 = local write "VPI C1"(w803) -> ()
                    n256 = local write "VPI C2"(w803) -> ()
                    n257 = local write "VPI C3"(w803) -> ()
                    n258 = local write "% Delta C"(w803) -> ()
                    n259 = local write "40V_3"(w803) -> ()
                    n260 = local write "40V_2"(w803) -> ()
                    n261 = local write "40V_1"(w803) -> ()
                  }
                }
                n262 = call "Delay T4.vi"("milliseconds to wait"=u32 50, "error in (no error)"=w733) -> ("error out"=w686:errorcluster)  [unwired: 9 in]
                n263 = for {
                  tunnel: [w762] -> w744
                  tunnel: [w761] -> w707
                  tunnel: w705 -> [w760]
                  tunnel: w693 -> [w759]
                  tunnel: w686 -> [w755]
                  tunnel: string[] ["0702013B3B3B", "070201000000"] -> [w751] mode=indexing
                  tunnel: [w750] -> w689 mode=indexing
                  n264 = call "WSVCAP SHL Host TL RFFE Write - Multiple DUTs - Common Data.vi"("Data Out"=w751, "error in"=w755, "Log (T)"=w760) -> ("error out"=w756:errorcluster)  [unwired: 12 in]
                  n265 = local read "IDD Brd(uA)"() -> (w752:string)
                  n266 = call "Delay T4.vi"("milliseconds to wait"=u32 100, "error in (no error)"=w756) -> ("error out"=w757:errorcluster)  [unwired: 9 in]
                  n267 = call "Ke2000 Single Reading.vi"("error in (no error)"=w757, "VISA resource name"=w759) -> ("error out"=w754:errorcluster, "VISA resource name out"=w762:refnum<visa-resource-name>, "uA"=w753:string)  [unwired: 5 in, 2 out]
                  n268 = call "Substration.vi"("error in (no error)"=w754, "Input2"=w752, "Input1"=w753) -> ("error out"=w761:errorcluster, "In1 - In2"=w750:string)  [unwired: 7 in]
                }
                n269 = Index Array(array=w689, index=1) -> (element=w688:string)
                n270 = Index Array(array=w689, index=0) -> (element=w691:string)
                n271 = local read "Clock Rate (Hz)"() -> (w734:dbl)
                n272 = call "Multi Dut Cmd_Header Setting.vi"("WS1050/51"="WS1050/51", "Cmin/Act"="Cmin/Act", "Test Seq"="Test Sequences", "error in (no error)"=w703) -> ("Name 1"=w701:string[], "Name 2"=w700:string[], "Name Header"=w698:string[], "Name 3"=w699:string[], "Cmd 3"=w695:string[], "Cmd 1"=w697:string[], "Cmd 2"=w696:string[], "error out"=w704:errorcluster)  [unwired: 2 in, 2 out]
              }
              frame #1 {
                w1046 = FALSE ("Log (T)")
                n273 = call "WSVCAP SHL Host TL RFFE Configure.vi"("RFFE Slave Address"=w1057, "Clock Rate (Hz)"=w1055, "error in"=w1047) -> ("Actual Rate (Hz)"=w1067:dbl, "error out"=w1053:errorcluster)  [unwired: 11 in]
                n274 = local write "AR  Measurent(Hz)"(w1067) -> ()
                n275 = Array Size(array=w1058) -> (size(s)=w1070:i32)
                n276 = case shown="2" w1040 {
                  tunnel: w1070 -> [w1079 w1111 w1143]
                  tunnel: w1064 -> [w1078 w1110 w1142]
                  tunnel: [w1077 w1109 w1141] -> w1060
                  tunnel: w1059 -> [w1076 w1108 w1140]
                  tunnel: w1058 -> [w1075 w1107 w1139]
                  tunnel: w1053 -> [w1074 w1106 w1138]
                  tunnel: [w1073 w1105 w1137] -> w1052
                  tunnel: w1046 -> [w1072 w1104 w1136]
                  tunnel: [w1071 w1103 w1135] -> w1041
                  frame 0, Default {
                    n277 = for {
                      N: w1079 -> [_]
                      tunnel: w1076 -> [w1098]
                      tunnel: w1078 -> [w1096]
                      tunnel: [w1095] -> w1077
                      tunnel: [w1091] -> w1071 mode=indexing
                      tunnel: w1075 -> [w1093]
                      tunnel: w1074 -> [w1081]
                      tunnel: [w1083] -> w1073
                      tunnel: w1072 -> [w1082]
                      i -> [w1090]
                      stop <- w1095 stop-if-true
                      n278 = Index Array(array=w1098, index=w1090) -> (element=w1094:string)
                      n279 = Index Array(array=w1093, index=w1090) -> (element=w1092:string)
                      n280 = local write "STATUS"(w1092) -> ()
                      n281 = call "WSVCAP SHL Host TL RFFE Write - Multiple DUTs - Common Data.vi"("Data Out"=w1094, "error in"=w1081, "Log (T)"=FALSE) -> ("error out"=w1085:errorcluster)  [unwired: 12 in]
                      n282 = call "Delay T4.vi"("milliseconds to wait"=u32 10, "error in (no error)"=w1085) -> ("error out"=w1089:errorcluster)  [unwired: 9 in]
                      n283 = call "WS1050 AD7747 READ 36 DUT.vi"("error in"=w1089, "Log (T)"=w1082, "DUT Mask Mode (All)"=WSVCAP_SHL_I2C_DUT_Mask_Mode_Enum."C1") -> ("error out"=w1087:errorcluster, "AD7747 Values"=w1088:string[][])  [unwired: 7 in]
                      n284 = for {
                        tunnel: w1088 -> [w1101] mode=indexing
                        tunnel: w1087 -> [w1102]
                        tunnel: [w1102] -> w1083
                        tunnel: [w1099] -> w1091 mode=indexing
                        n285 = Index Array(array=w1101, index=1) -> (element=w1099:string)
                      }
                      n286 = Unbundle By Name(w1083) -> ("status"=w1097:bool)
                      n287 = Or(x=w1097, y=w1096) -> (x .or. y?=w1095:bool)
                    }
                  }
                  frame 1 {
                    n288 = for {
                      N: w1111 -> [_]
                      tunnel: w1108 -> [w1130]
                      tunnel: w1110 -> [w1128]
                      tunnel: [w1127] -> w1109
                      tunnel: [w1123] -> w1103 mode=indexing
                      tunnel: w1107 -> [w1125]
                      tunnel: w1106 -> [w1113]
                      tunnel: [w1115] -> w1105
                      tunnel: w1104 -> [w1114]
                      i -> [w1122]
                      stop <- w1127 stop-if-true
                      n289 = Index Array(array=w1130, index=w1122) -> (element=w1126:string)
                      n290 = Index Array(array=w1125, index=w1122) -> (element=w1124:string)
                      n291 = local write "STATUS"(w1124) -> ()
                      n292 = call "WSVCAP SHL Host TL RFFE Write - Multiple DUTs - Common Data.vi"("Data Out"=w1126, "error in"=w1113, "Log (T)"=FALSE) -> ("error out"=w1117:errorcluster)  [unwired: 12 in]
                      n293 = call "Delay T4.vi"("milliseconds to wait"=u32 10, "error in (no error)"=w1117) -> ("error out"=w1121:errorcluster)  [unwired: 9 in]
                      n294 = call "WS1050 AD7747 READ 36 DUT.vi"("error in"=w1121, "Log (T)"=w1114, "DUT Mask Mode (All)"=WSVCAP_SHL_I2C_DUT_Mask_Mode_Enum."C2") -> ("error out"=w1119:errorcluster, "AD7747 Values"=w1120:string[][])  [unwired: 7 in]
                      n295 = for {
                        tunnel: w1120 -> [w1133] mode=indexing
                        tunnel: w1119 -> [w1134]
                        tunnel: [w1134] -> w1115
                        tunnel: [w1131] -> w1123 mode=indexing
                        n296 = Index Array(array=w1133, index=3) -> (element=w1131:string)
                      }
                      n297 = Unbundle By Name(w1115) -> ("status"=w1129:bool)
                      n298 = Or(x=w1129, y=w1128) -> (x .or. y?=w1127:bool)
                    }
                  }
                  frame 2 {
                    n299 = for {
                      N: w1143 -> [_]
                      tunnel: w1140 -> [w1162]
                      tunnel: w1142 -> [w1160]
                      tunnel: [w1159] -> w1141
                      tunnel: [w1155] -> w1135 mode=indexing
                      tunnel: w1139 -> [w1157]
                      tunnel: w1138 -> [w1145]
                      tunnel: [w1147] -> w1137
                      tunnel: w1136 -> [w1146]
                      i -> [w1154]
                      stop <- w1159 stop-if-true
                      n300 = Index Array(array=w1162, index=w1154) -> (element=w1158:string)
                      n301 = Index Array(array=w1157, index=w1154) -> (element=w1156:string)
                      n302 = local write "STATUS"(w1156) -> ()
                      n303 = call "WSVCAP SHL Host TL RFFE Write - Multiple DUTs - Common Data.vi"("Data Out"=w1158, "error in"=w1145, "Log (T)"=FALSE) -> ("error out"=w1149:errorcluster)  [unwired: 12 in]
                      n304 = call "Delay T4.vi"("milliseconds to wait"=u32 10, "error in (no error)"=w1149) -> ("error out"=w1153:errorcluster)  [unwired: 9 in]
                      n305 = call "WS1050 AD7747 READ 36 DUT.vi"("error in"=w1153, "Log (T)"=w1146, "DUT Mask Mode (All)"=WSVCAP_SHL_I2C_DUT_Mask_Mode_Enum."C3") -> ("error out"=w1151:errorcluster, "AD7747 Values"=w1152:string[][])  [unwired: 7 in]
                      n306 = for {
                        tunnel: w1152 -> [w1165] mode=indexing
                        tunnel: w1151 -> [w1166]
                        tunnel: [w1166] -> w1147
                        tunnel: [w1163] -> w1155 mode=indexing
                        n307 = Index Array(array=w1165, index=5) -> (element=w1163:string)
                      }
                      n308 = Unbundle By Name(w1147) -> ("status"=w1161:bool)
                      n309 = Or(x=w1161, y=w1160) -> (x .or. y?=w1159:bool)
                    }
                  }
                }
                n310 = Transpose 2D Array(2D array=w1041) -> (transposed array=w1051:string[][])
                "40V_1" <- w1051
                "NOM IDD ON (uA)" <- w1062
                "NOM IDD OFF(uA)" <- w1061
              }
              frame #2 {
                n311 = Array Size(array=w1185) -> (size(s)=w1186:i32)
                n312 = case shown="0, 2, Default" w1169 {
                  tunnel: w1186 -> [w1203 w1235]
                  tunnel: w1185 -> [w1202 w1234]
                  tunnel: w1184 -> [w1201 w1233]
                  tunnel: w1183 -> [w1200 w1232]
                  tunnel: [w1199 w1231] -> w1182
                  tunnel: [w1198 w1230] -> w1180
                  tunnel: w1178 -> [w1197 w1229]
                  tunnel: w1172 -> [w1196 w1228]
                  tunnel: [w1195 w1227] -> w1170
                  frame 0, 2, Default {
                    n313 = for {
                      N: w1203 -> [_]
                      tunnel: w1201 -> [w1222]
                      tunnel: w1200 -> [w1220]
                      tunnel: [w1219] -> w1199
                      tunnel: [w1215] -> w1195 mode=indexing
                      tunnel: w1202 -> [w1217]
                      tunnel: w1197 -> [w1205]
                      tunnel: [w1207] -> w1198
                      tunnel: w1196 -> [w1206]
                      i -> [w1214]
                      stop <- w1219 stop-if-true
                      n314 = Index Array(array=w1222, index=w1214) -> (element=w1218:string)
                      n315 = Index Array(array=w1217, index=w1214) -> (element=w1216:string)
                      n316 = call "WSVCAP SHL Host TL RFFE Write - Multiple DUTs - Common Data.vi"("Data Out"=w1218, "error in"=w1205, "Log (T)"=FALSE) -> ("error out"=w1209:errorcluster)  [unwired: 12 in]
                      n317 = local write "STATUS"(w1216) -> ()
                      n318 = call "Delay T4.vi"("milliseconds to wait"=u32 10, "error in (no error)"=w1209) -> ("error out"=w1213:errorcluster)  [unwired: 9 in]
                      n319 = call "WS1050 AD7747 READ 36 DUT.vi"("error in"=w1213, "Log (T)"=w1206, "DUT Mask Mode (All)"=WSVCAP_SHL_I2C_DUT_Mask_Mode_Enum."C2") -> ("error out"=w1211:errorcluster, "AD7747 Values"=w1212:string[][])  [unwired: 7 in]
                      n320 = for {
                        tunnel: w1212 -> [w1225] mode=indexing
                        tunnel: w1211 -> [w1226]
                        tunnel: [w1226] -> w1207
                        tunnel: [w1223] -> w1215 mode=indexing
                        n321 = Index Array(array=w1225, index=3) -> (element=w1223:string)
                      }
                      n322 = Unbundle By Name(w1207) -> ("status"=w1221:bool)
                      n323 = Or(x=w1221, y=w1220) -> (x .or. y?=w1219:bool)
                    }
                  }
                  frame 1 {
                    n324 = for {
                      N: w1235 -> [_]
                      tunnel: w1233 -> [w1254]
                      tunnel: w1232 -> [w1252]
                      tunnel: [w1251] -> w1231
                      tunnel: [w1247] -> w1227 mode=indexing
                      tunnel: w1234 -> [w1249]
                      tunnel: w1229 -> [w1237]
                      tunnel: [w1239] -> w1230
                      tunnel: w1228 -> [w1238]
                      i -> [w1246]
                      stop <- w1251 stop-if-true
                      n325 = Index Array(array=w1254, index=w1246) -> (element=w1250:string)
                      n326 = Index Array(array=w1249, index=w1246) -> (element=w1248:string)
                      n327 = call "WSVCAP SHL Host TL RFFE Write - Multiple DUTs - Common Data.vi"("Data Out"=w1250, "error in"=w1237, "Log (T)"=FALSE) -> ("error out"=w1241:errorcluster)  [unwired: 12 in]
                      n328 = local write "STATUS"(w1248) -> ()
                      n329 = call "Delay T4.vi"("milliseconds to wait"=u32 10, "error in (no error)"=w1241) -> ("error out"=w1245:errorcluster)  [unwired: 9 in]
                      n330 = call "WS1050 AD7747 READ 36 DUT.vi"("error in"=w1245, "Log (T)"=w1238, "DUT Mask Mode (All)"=WSVCAP_SHL_I2C_DUT_Mask_Mode_Enum."C1") -> ("error out"=w1243:errorcluster, "AD7747 Values"=w1244:string[][])  [unwired: 7 in]
                      n331 = for {
                        tunnel: w1244 -> [w1257] mode=indexing
                        tunnel: w1243 -> [w1258]
                        tunnel: [w1258] -> w1239
                        tunnel: [w1255] -> w1247 mode=indexing
                        n332 = Index Array(array=w1257, index=1) -> (element=w1255:string)
                      }
                      n333 = Unbundle By Name(w1239) -> ("status"=w1253:bool)
                      n334 = Or(x=w1253, y=w1252) -> (x .or. y?=w1251:bool)
                    }
                  }
                }
                n335 = Transpose 2D Array(2D array=w1170) -> (transposed array=w1179:string[][])
                "40V_2" <- w1179
              }
              frame #3 {
                n336 = Array Size(array=w1277) -> (size(s)=w1278:i32)
                n337 = case shown="2" w1262 {
                  tunnel: w1278 -> [w1296 w1328]
                  tunnel: w1277 -> [w1295 w1327]
                  tunnel: w1276 -> [w1294 w1326]
                  tunnel: w1275 -> [w1293 w1325]
                  tunnel: [w1292 w1324] -> w1274
                  tunnel: w1269 -> [w1291 w1323]
                  tunnel: [w1290 w1322] -> w1261
                  tunnel: w1265 -> [w1289 w1321]
                  tunnel: [w1288 w1320] -> w1263
                  frame 0, 1, Default {
                    n338 = for {
                      N: w1296 -> [_]
                      tunnel: w1294 -> [w1315]
                      tunnel: w1293 -> [w1313]
                      tunnel: [w1312] -> w1292
                      tunnel: [w1308] -> w1288 mode=indexing
                      tunnel: w1295 -> [w1310]
                      tunnel: w1291 -> [w1298]
                      tunnel: [w1300] -> w1290
                      tunnel: w1289 -> [w1299]
                      i -> [w1307]
                      stop <- w1312 stop-if-true
                      n339 = Index Array(array=w1315, index=w1307) -> (element=w1311:string)
                      n340 = Index Array(array=w1310, index=w1307) -> (element=w1309:string)
                      n341 = local write "STATUS"(w1309) -> ()
                      n342 = call "WSVCAP SHL Host TL RFFE Write - Multiple DUTs - Common Data.vi"("Data Out"=w1311, "error in"=w1298, "Log (T)"=FALSE) -> ("error out"=w1302:errorcluster)  [unwired: 12 in]
                      n343 = call "Delay T4.vi"("milliseconds to wait"=u32 10, "error in (no error)"=w1302) -> ("error out"=w1306:errorcluster)  [unwired: 9 in]
                      n344 = call "WS1050 AD7747 READ 36 DUT.vi"("error in"=w1306, "Log (T)"=w1299, "DUT Mask Mode (All)"=WSVCAP_SHL_I2C_DUT_Mask_Mode_Enum."C3") -> ("error out"=w1304:errorcluster, "AD7747 Values"=w1305:string[][])  [unwired: 7 in]
                      n345 = for {
                        tunnel: w1305 -> [w1318] mode=indexing
                        tunnel: w1304 -> [w1319]
                        tunnel: [w1319] -> w1300
                        tunnel: [w1316] -> w1308 mode=indexing
                        n346 = Index Array(array=w1318, index=5) -> (element=w1316:string)
                      }
                      n347 = Unbundle By Name(w1300) -> ("status"=w1314:bool)
                      n348 = Or(x=w1314, y=w1313) -> (x .or. y?=w1312:bool)
                    }
                  }
                  frame 2 {
                    n349 = for {
                      N: w1328 -> [_]
                      tunnel: w1326 -> [w1347]
                      tunnel: w1325 -> [w1345]
                      tunnel: [w1344] -> w1324
                      tunnel: [w1340] -> w1320 mode=indexing
                      tunnel: w1327 -> [w1342]
                      tunnel: w1323 -> [w1330]
                      tunnel: [w1332] -> w1322
                      tunnel: w1321 -> [w1331]
                      i -> [w1339]
                      stop <- w1344 stop-if-true
                      n350 = Index Array(array=w1347, index=w1339) -> (element=w1343:string)
                      n351 = Index Array(array=w1342, index=w1339) -> (element=w1341:string)
                      n352 = local write "STATUS"(w1341) -> ()
                      n353 = call "WSVCAP SHL Host TL RFFE Write - Multiple DUTs - Common Data.vi"("Data Out"=w1343, "error in"=w1330, "Log (T)"=FALSE) -> ("error out"=w1334:errorcluster)  [unwired: 12 in]
                      n354 = call "Delay T4.vi"("milliseconds to wait"=u32 10, "error in (no error)"=w1334) -> ("error out"=w1338:errorcluster)  [unwired: 9 in]
                      n355 = call "WS1050 AD7747 READ 36 DUT.vi"("error in"=w1338, "Log (T)"=w1331, "DUT Mask Mode (All)"=WSVCAP_SHL_I2C_DUT_Mask_Mode_Enum."C1") -> ("error out"=w1336:errorcluster, "AD7747 Values"=w1337:string[][])  [unwired: 7 in]
                      n356 = for {
                        tunnel: w1337 -> [w1350] mode=indexing
                        tunnel: w1336 -> [w1351]
                        tunnel: [w1351] -> w1332
                        tunnel: [w1348] -> w1340 mode=indexing
                        n357 = Index Array(array=w1350, index=1) -> (element=w1348:string)
                      }
                      n358 = Unbundle By Name(w1332) -> ("status"=w1346:bool)
                      n359 = Or(x=w1346, y=w1345) -> (x .or. y?=w1344:bool)
                    }
                  }
                }
                n360 = Transpose 2D Array(2D array=w1263) -> (transposed array=w1270:string[][])
                "40V_3" <- w1270
              }
              frame #4 {
                # "VPI Testing @ 35V"
                n361 = call "WS1050 Delta C Calculation.vi"("error in (no error)"=w1392, "DCap Target(pF)"=w1391, "Input"=w1394) -> ("error out"=w1389:errorcluster, "Total Bank Delta C(pF)"=w1382:string[], "% Bank DeltaC"=w1386:string[])  [unwired: 4 in, 2 out]
                n362 = call "WS1050 Delta C Calculation.vi"("error in (no error)"=w1392, "DCap Target(pF)"=w1391, "Input"=w1393) -> ("error out"=w1390:errorcluster, "Total Bank Delta C(pF)"=w1381:string[], "% Bank DeltaC"=w1384:string[])  [unwired: 4 in, 2 out]
                n363 = call "WS1050 Delta C Calculation.vi"("error in (no error)"=w1392, "DCap Target(pF)"=w1391, "Input"=w1385) -> ("error out"=w1388:errorcluster, "Total Bank Delta C(pF)"=w1380:string[], "% Bank DeltaC"=w1383:string[])  [unwired: 4 in, 2 out]
                n364 = Merge Errors(w1389, w1390, w1388) -> (w1387:errorcluster)
                n365 = case shown="1, Default" w1395 {
                  tunnel: w1387 -> [w1425 w1433]
                  tunnel: [w1425 w1433] -> w1354
                  tunnel: w1386 -> [w1421 w1429]
                  tunnel: w1384 -> [w1420 w1428]
                  tunnel: w1383 -> [w1419 w1427]
                  tunnel: w1382 -> [w1424 w1432]
                  tunnel: [w1424 w1432] -> w1379
                  tunnel: w1381 -> [w1423 w1431]
                  tunnel: [w1423 w1431] -> w1378
                  tunnel: w1380 -> [w1422 w1430]
                  tunnel: [w1422 w1430] -> w1377
                  frame 0 {
                    n366 = Build Array(w1421, w1420, w1419) -> (→"% Delta C_T0":string[][])
                  }
                  frame 1, Default {
                    n367 = Build Array(w1429, w1428, w1427) -> (→"% Delta C":string[][])
                  }
                }
                "Total Delta C1(pF)" <- w1379
                "Total Delta C2(pF)" <- w1378
                "Total Delta C3(pF)" <- w1377
                n368 = call "WS1050_51 VPI Header.vi"("VPI Name"="VPI Name", "VPI_Cmd"="VPI_Cmd", "Cmin/Act"=w1352, "WS1050/51"=w1363, "error in (no error)"=w1364) -> ("VPI_1"=w1362:string[], "VPI_2"=w1360:string[], "VPI Header"=w1361:string[], "VPI_3"=w1359:string[], "Cmd_3"=w1356:string[], "Cmd_1"=w1358:string[], "Cmd_2"=w1357:string[], "error out"=w1355:errorcluster)  [unwired: 3 in]
                n369 = Merge Errors(w1355, w1354) -> (w1353:errorcluster)
                n370 = case shown="True" w1369 {
                  tunnel: w1409 -> [w1440 w1478]
                  tunnel: [w1436 w1456] -> w1373
                  tunnel: [w1434 w1480] -> w1408
                  tunnel: [w1434 w1464] -> w1407
                  tunnel: [w1440 w1462] -> w1405
                  tunnel: w1402 -> [w1442 w1479]
                  tunnel: [w1442 w1479] -> w1401
                  tunnel: w1358 -> [_ w1477]
                  tunnel: w1357 -> [_ w1471]
                  tunnel: w1356 -> [_ w1466]
                  tunnel: [w1434 w1476] -> w1398
                  tunnel: w1362 -> [w1439 w1474]
                  tunnel: w1360 -> [_ w1472]
                  tunnel: w1359 -> [_ w1467]
                  tunnel: ["NA" ("string") w1461] -> w1375
                  tunnel: w1353 -> [w1437 w1453]
                  frame False {
                    n371 = Array Size(array=w1439) -> (size(s)=w1438:i32)
                    n372 = for {
                      N: w1438 -> [_]
                      tunnel: [w1444] -> w1435 mode=indexing
                      tunnel: w1437 -> [w1443]
                      tunnel: [w1443] -> w1436
                      n373 = for {
                        N: 36 -> [_]
                        tunnel: ["na"] -> w1444 mode=indexing
                      }
                    }
                    n374 = Transpose 2D Array(2D array=w1435) -> (transposed array=w1434:string[][])
                    n375 = local write "VPI C1"(w1434) -> ()
                    n376 = local write "VPI C2"(w1434) -> ()
                    n377 = local write "VPI C3"(w1434) -> ()
                  }
                  frame True {
                    w1455 = FALSE ("Log (T)")
                    # "Set CP to 35V"
                    n378 = call "WSVCAP SHL Host TL RFFE Write - Multiple DUTs - Common Data.vi"("Data Out"="074820", "error in"=w1453, "Log (T)"=w1455) -> ("error out"=w1451:errorcluster)  [unwired: 12 in]
                    n379 = call "Delay T4.vi"("milliseconds to wait"=u32 10, "error in (no error)"=w1451) -> ("error out"=w1457:errorcluster)  [unwired: 9 in]
                    n380 = case shown="3" "CP VPI" {
                      selector: "CP VPI" -> [w1485 w1490 w1495 w1499]
                      tunnel: string[] ["07476F", "074776", "074765", "074769", "07477B"] -> [w1486 w1491 w1496 w1501]
                      tunnel: [w1484 w1489 w1494 w1500] -> w1449
                      tunnel: [w1482 w1487 w1492 w1497] -> w1448
                      tunnel: ["35" ("string") "27.5" ("string") "30.5" ("string") "40.25" ("string")] -> w1461
                      tunnel: w1457 -> [w1482 w1487 w1492 w1497]
                      frame 0, Default {
                        n381 = Index Array(array=w1486, index=w1485) -> (element=w1484:string)
                      }
                      frame 2 {
                        n382 = Index Array(array=w1491, index=w1490) -> (element=w1489:string)
                      }
                      frame 3 {
                        n383 = Index Array(array=w1496, index=w1495) -> (element=w1494:string)
                      }
                      frame 1 {
                        n384 = Index Array(array=w1501, index=w1499) -> (element=w1500:string)
                      }
                    }
                    n385 = Array Size(array=w1474) -> (size(s)=w1481:i32)
                    n386 = call "WSVCAP SHL Host TL RFFE Write - Multiple DUTs - Common Data.vi"("Data Out"=w1449, "error in"=w1448, "Log (T)"=w1455) -> ("error out"=w1460:errorcluster)  [unwired: 12 in]
                    n387 = for {
                      N: w1481 -> [_]
                      tunnel: w1477 -> [w1566]
                      tunnel: w1478 -> [w1564]
                      tunnel: [w1563] -> w1470
                      tunnel: [w1561] -> w1475 mode=indexing
                      tunnel: w1474 -> [w1560]
                      tunnel: w1460 -> [w1549]
                      tunnel: [w1551] -> w1459
                      i -> [w1559]
                      stop <- w1563 stop-if-true
                      n388 = Index Array(array=w1566, index=w1559) -> (element=w1562:string)
                      n389 = Index Array(array=w1560, index=w1559) -> (element=w1558:string)
                      n390 = local write "STATUS"(w1558) -> ()
                      n391 = call "WSVCAP SHL Host TL RFFE Write - Multiple DUTs - Common Data.vi"("Data Out"=w1562, "error in"=w1549, "Log (T)"=FALSE) -> ("error out"=w1557:errorcluster)  [unwired: 12 in]
                      n392 = call "Delay T4.vi"("milliseconds to wait"=u32 10, "error in (no error)"=w1557) -> ("error out"=w1553:errorcluster)  [unwired: 9 in]
                      n393 = call "WS1050 AD7747 READ 36 DUT.vi"("error in"=w1553, "Log (T)"=FALSE, "DUT Mask Mode (All)"=WSVCAP_SHL_I2C_DUT_Mask_Mode_Enum."C1") -> ("error out"=w1555:errorcluster, "AD7747 Values"=w1554:string[][])  [unwired: 7 in]
                      n394 = for {
                        tunnel: [w1569] -> w1561 mode=indexing
                        tunnel: w1555 -> [w1568]
                        tunnel: [w1568] -> w1551
                        tunnel: w1554 -> [w1567] mode=indexing
                        n395 = Index Array(array=w1567, index=1) -> (element=w1569:string)
                      }
                      n396 = Unbundle By Name(w1551) -> ("status"=w1565:bool)
                      n397 = Or(x=w1565, y=w1564) -> (x .or. y?=w1563:bool)
                    }
                    n398 = Transpose 2D Array(2D array=w1475) -> (transposed array=w1480:string[][])
                    "VPI C1" <- w1480
                    n399 = Array Size(array=w1472) -> (size(s)=w1473:i32)
                    n400 = for {
                      N: w1473 -> [_]
                      tunnel: w1471 -> [w1543]
                      tunnel: w1470 -> [w1541]
                      tunnel: [w1540] -> w1463
                      tunnel: [w1538] -> w1469 mode=indexing
                      tunnel: w1472 -> [w1537]
                      tunnel: w1459 -> [w1526]
                      tunnel: [w1528] -> w1458
                      i -> [w1536]
                      stop <- w1540 stop-if-true
                      n401 = Index Array(array=w1543, index=w1536) -> (element=w1539:string)
                      n402 = Index Array(array=w1537, index=w1536) -> (element=w1535:string)
                      n403 = call "WSVCAP SHL Host TL RFFE Write - Multiple DUTs - Common Data.vi"("Data Out"=w1539, "error in"=w1526, "Log (T)"=FALSE) -> ("error out"=w1534:errorcluster)  [unwired: 12 in]
                      n404 = local write "STATUS"(w1535) -> ()
                      n405 = call "Delay T4.vi"("milliseconds to wait"=u32 10, "error in (no error)"=w1534) -> ("error out"=w1530:errorcluster)  [unwired: 9 in]
                      n406 = call "WS1050 AD7747 READ 36 DUT.vi"("error in"=w1530, "Log (T)"=FALSE, "DUT Mask Mode (All)"=WSVCAP_SHL_I2C_DUT_Mask_Mode_Enum."C2") -> ("error out"=w1532:errorcluster, "AD7747 Values"=w1531:string[][])  [unwired: 7 in]
                      n407 = for {
                        tunnel: [w1546] -> w1538 mode=indexing
                        tunnel: w1532 -> [w1545]
                        tunnel: [w1545] -> w1528
                        tunnel: w1531 -> [w1544] mode=indexing
                        n408 = Index Array(array=w1544, index=3) -> (element=w1546:string)
                      }
                      n409 = Unbundle By Name(w1528) -> ("status"=w1542:bool)
                      n410 = Or(x=w1542, y=w1541) -> (x .or. y?=w1540:bool)
                    }
                    n411 = Transpose 2D Array(2D array=w1469) -> (transposed array=w1476:string[][])
                    "VPI C2" <- w1476
                    n412 = Array Size(array=w1467) -> (size(s)=w1468:i32)
                    n413 = for {
                      N: w1468 -> [_]
                      tunnel: w1466 -> [w1520]
                      tunnel: w1463 -> [w1518]
                      tunnel: [w1517] -> w1462
                      tunnel: [w1515] -> w1465 mode=indexing
                      tunnel: w1467 -> [w1514]
                      tunnel: w1458 -> [w1503]
                      tunnel: [w1505] -> w1456
                      i -> [w1513]
                      stop <- w1517 stop-if-true
                      n414 = Index Array(array=w1520, index=w1513) -> (element=w1516:string)
                      n415 = Index Array(array=w1514, index=w1513) -> (element=w1512:string)
                      n416 = call "WSVCAP SHL Host TL RFFE Write - Multiple DUTs - Common Data.vi"("Data Out"=w1516, "error in"=w1503, "Log (T)"=FALSE) -> ("error out"=w1511:errorcluster)  [unwired: 12 in]
                      n417 = local write "STATUS"(w1512) -> ()
                      n418 = call "Delay T4.vi"("milliseconds to wait"=u32 10, "error in (no error)"=w1511) -> ("error out"=w1507:errorcluster)  [unwired: 9 in]
                      n419 = call "WS1050 AD7747 READ 36 DUT.vi"("error in"=w1507, "Log (T)"=FALSE, "DUT Mask Mode (All)"=WSVCAP_SHL_I2C_DUT_Mask_Mode_Enum."C3") -> ("error out"=w1509:errorcluster, "AD7747 Values"=w1508:string[][])  [unwired: 7 in]
                      n420 = for {
                        tunnel: [w1523] -> w1515 mode=indexing
                        tunnel: w1509 -> [w1522]
                        tunnel: [w1522] -> w1505
                        tunnel: w1508 -> [w1521] mode=indexing
                        n421 = Index Array(array=w1521, index=5) -> (element=w1523:string)
                      }
                      n422 = Unbundle By Name(w1505) -> ("status"=w1519:bool)
                      n423 = Or(x=w1519, y=w1518) -> (x .or. y?=w1517:bool)
                    }
                    n424 = Transpose 2D Array(2D array=w1465) -> (transposed array=w1464:string[][])
                    "VPI C3" <- w1464
                  }
                }
                n425 = Insert Into Array(array=w1397, new element=w1361) -> (w1396:string[])  [unwired: 1 in]
                n426 = case shown="True" w1374 {
                  tunnel: w1373 -> [w1411 w1416]
                  tunnel: [w1412 w1415] -> w1372
                  frame False {
                    n427 = call "WSVCAP SHL Host TL RFFE Write - Multiple DUTs - Common Data.vi"("Data Out"="074820", "error in"=w1411, "Log (T)"=FALSE) -> ("error out"=w1412:errorcluster)  [unwired: 12 in]
                  }
                  frame True {
                    n428 = call "WSVCAP SHL Host TL RFFE Write - Multiple DUTs - Common Data.vi"("Data Out"="074800", "error in"=w1416, "Log (T)"=FALSE) -> ("error out"=w1415:errorcluster)  [unwired: 12 in]
                  }
                }
                n429 = call "Delay T4.vi"("milliseconds to wait"=u32 10, "error in (no error)"=w1372) -> ("error out"=w1371:errorcluster)  [unwired: 9 in]
              }
              frame #5 {
                # "VSA Testing"
                n430 = case shown="False" w1571 {
                  tunnel: w1610 -> [w1622 w1636]
                  tunnel: [w1621 w1635] -> w1584
                  tunnel: [w1626 w1642] -> w1600
                  tunnel: w1601 -> [w1626 w1641]
                  tunnel: [w1623 w1639] -> w1589
                  tunnel: [w1623 w1638] -> w1586
                  tunnel: [w1623 w1637] -> w1583
                  tunnel: [w1624 w1640] -> w1590
                  frame False {
                    n431 = for {
                      tunnel: dbl[] [0.0, 0.0, 0.0] -> [w1631] mode=indexing
                      tunnel: [w1630] -> w1624 mode=indexing
                      tunnel: [w1628] -> w1623 mode=indexing
                      tunnel: w1622 -> [w1627]
                      tunnel: [w1627] -> w1621
                      w1629 = 36
                      n432 = Number To Fractional String(number=w1631) -> (F-format string=w1632:string)  [unwired: 3 in]
                      n433 = for {
                        N: w1629 -> [_]
                        tunnel: w1632 -> [w1634]
                        tunnel: [w1634] -> w1630 mode=indexing
                      }
                      n434 = for {
                        N: w1629 -> [_]
                        tunnel: ["na"] -> w1628 mode=indexing
                      }
                    }
                  }
                  frame True {
                    n435 = for {
                      tunnel: "VSA Voltage(V)" -> [w1666] mode=indexing
                      tunnel: [w1670] -> w1642
                      tunnel: w1641 -> [w1668]
                      tunnel: [w1667] -> w1639 mode=indexing
                      tunnel: [w1654] -> w1638 mode=indexing
                      tunnel: [w1663] -> w1640 mode=indexing
                      tunnel: [w1648] -> w1637 mode=indexing
                      tunnel: w1636 -> [w1647]
                      tunnel: [w1646] -> w1635
                      w1645 = FALSE ("Log (T)")
                      w1662 = u16 0 items=["Voltage", "Current"] ("Source Mode  (0: Voltage)")
                      n436 = call "Configure Output.vi"("Source Mode  (0: Voltage)"=w1662, "error in (no error)"=w1647, "Compliance  Level (0.1)"=0.1, "Output Level (0)"=w1666, "VISA resource name"=w1668) -> ("error out"=w1674:errorcluster, "VISA resource name out"=w1672:refnum<visa-resource-name>)  [unwired: 5 in]
                      n437 = Number To Fractional String(number=w1666) -> (F-format string=w1665:string)  [unwired: 3 in]
                      n438 = call "Enable Output.vi"("error in (no error)"=w1674, "Enable Output (T: Enable)"=TRUE, "VISA resource name"=w1672) -> ("error out"=w1675:errorcluster, "VISA resource name out"=w1670:refnum<visa-resource-name>)  [unwired: 7 in]
                      n439 = call "Delay T4.vi"("milliseconds to wait"=u32 10, "error in (no error)"=w1675) -> ("error out"=w1661:errorcluster)  [unwired: 9 in]
                      n440 = call "WS1050 AD7747 READ 36 DUT.vi"("error in"=w1661, "Log (T)"=w1645, "DUT Mask Mode (All)"=WSVCAP_SHL_I2C_DUT_Mask_Mode_Enum."C1") -> ("error out"=w1658:errorcluster, "AD7747 Values"=w1660:string[][])  [unwired: 7 in]
                      n441 = for {
                        tunnel: w1660 -> [w1686] mode=indexing
                        tunnel: [w1687] -> w1667 mode=indexing
                        tunnel: w1658 -> [w1685]
                        tunnel: [w1685] -> w1657
                        n442 = Index Array(array=w1686, index=1) -> (element=w1687:string)
                      }
                      n443 = for {
                        N: 36 -> [_]
                        tunnel: w1665 -> [w1684]
                        tunnel: [w1684] -> w1663 mode=indexing
                      }
                      n444 = call "WS1050 AD7747 READ 36 DUT.vi"("error in"=w1657, "Log (T)"=w1645, "DUT Mask Mode (All)"=WSVCAP_SHL_I2C_DUT_Mask_Mode_Enum."C2") -> ("error out"=w1655:errorcluster, "AD7747 Values"=w1653:string[][])  [unwired: 7 in]
                      n445 = for {
                        tunnel: w1653 -> [w1681] mode=indexing
                        tunnel: [w1682] -> w1654 mode=indexing
                        tunnel: w1655 -> [w1680]
                        tunnel: [w1680] -> w1652
                        n446 = Index Array(array=w1681, index=3) -> (element=w1682:string)
                      }
                      n447 = call "WS1050 AD7747 READ 36 DUT.vi"("error in"=w1652, "Log (T)"=w1645, "DUT Mask Mode (All)"=WSVCAP_SHL_I2C_DUT_Mask_Mode_Enum."C3") -> ("error out"=w1650:errorcluster, "AD7747 Values"=w1649:string[][])  [unwired: 7 in]
                      n448 = for {
                        tunnel: w1649 -> [w1677] mode=indexing
                        tunnel: [w1678] -> w1648 mode=indexing
                        tunnel: w1650 -> [w1676]
                        tunnel: [w1676] -> w1646
                        n449 = Index Array(array=w1677, index=5) -> (element=w1678:string)
                      }
                    }
                    n450 = local write "STATUS"("VSA Testing...." ("STATUS")) -> ()
                  }
                }
                n451 = Transpose 2D Array(2D array=w1590) -> (transposed array=w1588:string[][])
                n452 = Transpose 2D Array(2D array=w1589) -> (transposed array=w1587:string[][])
                n453 = Transpose 2D Array(2D array=w1586) -> (transposed array=w1585:string[][])
                n454 = Transpose 2D Array(2D array=w1583) -> (transposed array=w1582:string[][])
                n455 = call "WS1050_VSA_Convert_Data.vi"("VSA_C3"=w1582, "error in (no error)"=w1584, "VSA_C2"=w1585, "VSA_C1"=w1587, "Voltage"=w1588) -> ("error out"=w1581:errorcluster, "VSA_V3"=w1578:string[][], "VSA_V2"=w1579:string[][], "VSA_V1"=w1580:string[][])  [unwired: 3 in]
                "VSA_V1" <- w1580
                "VSA_V2" <- w1579
                "VSA_V3" <- w1578
                n456 = case shown="True" w1571 {
                  tunnel: w1600 -> [w1614 w1620]
                  tunnel: [w1614 w1619] -> w1599
                  tunnel: w1581 -> [w1613 w1618]
                  tunnel: [w1613 w1615] -> w1598
                  frame False {
                  }
                  frame True {
                    w1616 = u16 0 items=["Voltage", "Current"] ("Source Mode  (0: Voltage)")
                    n457 = call "Configure Output.vi"("Source Mode  (0: Voltage)"=w1616, "error in (no error)"=w1618, "Output Level (0)"=0.0, "VISA resource name"=w1620) -> ("error out"=w1615:errorcluster, "VISA resource name out"=w1619:refnum<visa-resource-name>)  [unwired: 6 in]
                  }
                }
                n458 = call "Delay T4.vi"("milliseconds to wait"=u32 50, "error in (no error)"=w1598) -> ("error out"=w1597:errorcluster)  [unwired: 9 in]
              }
              frame #6 {
                # "Handshake Check and EFuse Readback"
                n459 = Or(x=w1697, y=w1707) -> (x .or. y?=w1706:bool)
                n460 = Add(x=w1719, y=w1718) -> (x+y=w1705:u64)
                n461 = case shown="True" w1706 {
                  tunnel: w1732 -> [w1745 _]
                  tunnel: w1731 -> [w1744 w1750]
                  tunnel: [w1743 w1750] -> w1730
                  tunnel: w1729 -> [w1742 _]
                  tunnel: w1728 -> [w1741 _]
                  tunnel: w1727 -> [w1740 _]
                  tunnel: [w1736 w1749] -> w1726
                  tunnel: [w1735 w1749] -> w1721
                  tunnel: w1705 -> [w1734 _]
                  tunnel: w1712 -> [w1733 _]
                  frame False {
                    n462 = call "WS1050_36DUT_Handshake Check R1_Record All Regs Ver1.0.vi"("file path (use dialog)"=w1745, "Reg1_Bit Cntrl"="Reg1_Bit Cntrl", "File Name"=w1733, "SN"=w1740, "Loop"=w1734, "error"=w1744, "Lot #"=w1742, "Wafer #"=w1741) -> ("Pass/Fail"=→"EFuse Readback Status":bool[], "EFuse Read back"=w1735:string[], "Status"=w1736:string[], "error out"=w1743:errorcluster)  [unwired: 6 in, 2 out]
                    n463 = case shown="1, Default" w1734 {
                      tunnel: w1735 -> [w1746 w1747]
                      frame 0 {
                        "EFuse RB T0" <- w1746
                      }
                      frame 1, Default {
                        "Current EFuse Read back" <- w1747
                      }
                    }
                    n464 = local write "STATUS"("Hand Shake & EFuse Readback...." ("STATUS")) -> ()
                  }
                  frame True {
                    n465 = for {
                      N: 36 -> [_]
                      tunnel: ["na"] -> w1749 mode=indexing
                    }
                  }
                }
                n466 = Add(x=w1705, y=w1702) -> (x+y=w1703:u64)
                "TTCompleted" <- w1703
                n467 = Number To Engineering String(4:w1703) -> (0:w1717:string)  [unwired: 3 in]
                n468 = Build Array(w1716, w1714, w1713) -> (w1715:string[])
              }
              frame #7 {
                # "Save Data"
                n469 = Increment(x=w1762) -> (x+1=w1761:i32)
                n470 = local write "STATUS"("Saving Data...." ("STATUS")) -> ()
                n471 = Multiply(x=w1761, y=36) -> (x*y=w1756:i32)
                n472 = Path To String(path=w1766) -> (string=w1765:string)
                n473 = Bundle("Test Program"=w1798, "Comment"=w1797, "Data Out"=w1773, "Data Out"=w1772, "Data Out"=w1771, w1770, "Data Out"=w1769, "Data Out"=w1768, "string"=w1767, "Freq(Hz)"=w1754, "Board#"=w1752) -> (w1753:T8)  [unwired: 1 in]
                n474 = case shown="True" "Debug" {
                  tunnel: w1756 -> [w1805 w1808]
                  tunnel: [w1805 w1806] -> w1755
                  frame False {
                  }
                  frame True {
                    n475 = Multiply(x=w1808, y="No of Rows\nFrom Spread Sheet") -> (x*y=w1806:i32)
                  }
                }
                n476 = call "WS1050_36 DUT SData Ver1.0.vi"("TMN DC\\CAP Data Log File Path"=w1766, "Lot#"=w1800, "Total Delta C1(pF)"=w1776, "VSA_V1"=w1785, "Wafer#"=w1796, "File Name"=w1759, "Total Delta C2(pF)"=w1775, "error in"=w1803, "TP/Comment"=w1753, "EFuse"=w1790, "Data Output C3"=w1778, "Temperature"=w1782, "VSA_V2"=w1786, "VPI C3"=w1780, "Data Output C1"=w1793, "VPI C2"=w1779, "SN"=w1801, "R/W Status"=w1799, "Cap Header"=w1781, "HD/Cycles Completed"=w1789, "Data Output C2"=w1777, "VSA_V3"=w1784, "Current"=w1792, "VPI C1"=w1791, "Total Delta C3(pF)"=w1774) -> ("error out"=w1802:errorcluster)  [unwired: 2 in]
                n477 = Concatenate Strings(w1765, "\\" ("string"), w1759, "_Multi Socket Data.csv" ("string")) -> (w1764:string)
              }
              frame #8 {
                n478 = case shown="True" "Plot Delta Cmin" {
                  tunnel: w1814 -> [w1828 w1843]
                  tunnel: [w1828 w1839] -> w1813
                  tunnel: w1812 -> [_ w1835]
                  tunnel: w1810 -> [_ w1833]
                  frame False {
                  }
                  frame True {
                    w1829 = 2 items=["C1", "C2", "C3", "D_C1", "D_C2", "D_C3"] ("Bank")
                    w1830 = 1 items=["C1", "C2", "C3", "D_C1", "D_C2", "D_C3"] ("Bank")
                    w1831 = 0 items=["C1", "C2", "C3", "D_C1", "D_C2", "D_C3"] ("Bank")
                    n479 = String To Path(string=w1835) -> (path=w1834:path)
                    n480 = call "Delay T4.vi"("milliseconds to wait"=u32 50, "error in (no error)"=w1843) -> ("error out"=w1842:errorcluster)  [unwired: 9 in]
                    n481 = call "36DUT Plot From Spread Sheet.vi"("Plot"="Plot", "No of Rows"=w1833, "error in (no error)"=w1842, "Bank"=w1831, "file path (dialog if empty)"=w1834) -> ("error out"=w1837:errorcluster, "Delta C_Min Plot"=→"Min Plot_1":dbl[][])  [unwired: 5 in]
                    n482 = call "36DUT Plot From Spread Sheet.vi"("Plot"="Plot", "No of Rows"=w1833, "error in (no error)"=w1837, "Bank"=w1830, "file path (dialog if empty)"=w1834) -> ("error out"=w1838:errorcluster, "Delta C_Min Plot"=→"Min Plot_2":dbl[][])  [unwired: 5 in]
                    n483 = call "36DUT Plot From Spread Sheet.vi"("Plot"="Plot", "No of Rows"=w1833, "error in (no error)"=w1838, "Bank"=w1829, "file path (dialog if empty)"=w1834) -> ("error out"=w1839:errorcluster, "Delta C_Min Plot"=→"Min Plot_3":dbl[][])  [unwired: 5 in]
                  }
                }
                n484 = Get Date/Time In Seconds() -> (seconds since 1Jan1904=w1821:timestamp)
                n485 = Get Date/Time String(seconds (now)=w1821, want seconds? (F)=TRUE) -> (date string=→"date string":string, time string=→"Previous Time":string)  [unwired: 1 in]
                n486 = Greater Or Equal?(x=w1818, y="Set HD/Cycle \nto Complete") -> (x >= y?=w1825:bool)
                n487 = Greater Or Equal?(x=w1817, y="TTF Completed") -> (x >= y?=w1816:bool)
                "No of HD/Cycle\nCompleted" <- w1818
              }
            }
            n488 = Increment(x=w577) -> (x+1=→"Loop \ncompleted":i32)
            n489 = call "Delay T4.vi"("milliseconds to wait"=u32 10, "error in (no error)"=w464) -> ("error out"=w465:errorcluster)  [unwired: 9 in]
            n490 = Compound Arithmetic op=OR(w646, w547, w573) -> (w586:bool)
          }
          "Total Time" <- w409
          n491 = Increment(x=w407) -> (x+1=→"Run Loops":i32)
          n492 = local write "No of HD/Cycle\nCompleted"(u64 0 ("No of HD/Cycle\nCompleted")) -> ()
          n493 = Unbundle By Name(w399) -> ("status"=w413:bool)
          n494 = Compound Arithmetic op=OR(w413, w405, w404) -> (w395:bool)
        }
        n495 = for {
          tunnel: w291 -> [w1855]
          tunnel: w269 -> [w1854]
          tunnel: w320 -> [w1852] mode=indexing
          tunnel: [w1847] -> w289
          tunnel: [w1851] -> w319
          n496 = call "E3631A_Voltage Controller.vi"("VISA resource name"=w1854, "I_VDD(A)"=0.5, "Channel Controller"=w1852, "Voltage 1"=0.0, "Voltage 2"=3.3, "error in (no error)"=w1855, "I_3.3V (A)"=0.5) -> ("VISA resource name out"=w1851:refnum<visa-resource-name>, "error out"=w1848:errorcluster)  [unwired: 7 in]
          n497 = call "Delay T4.vi"("milliseconds to wait"=u32 100, "error in (no error)"=w1848) -> ("error out"=w1847:errorcluster)  [unwired: 9 in]
        }
        n498 = VISA Write(VISA resource name=w310, write buffer="SOUR:FUNC VOLT;VOLT:MODE FIX;RANG 100;LEV 0.0;:SENS:FUNC \"CURR\";CURR:PROT 60E-3;RANG 100E-3;:OUTP ON", error in (no error)=w291) -> (VISA resource name out=w308:refnum<visa-resource-name>, error out=w290:errorcluster)  [unwired: 1 out]
        n499 = Merge Errors(w289, w290) -> (w309:errorcluster)
      }
      frame True {
      }
    }
    n500 = local write "stop During HD/Cycles"(w70) -> ()
    n501 = Wait Until Next ms Multiple(millisecond multiple=u32 100) -> ()  [unwired: 1 out]
    n502 = Unbundle By Name(w71) -> ("status"=w89:bool)
    n503 = Or(x=w89, y=w80) -> (x .or. y?=w88:bool)
    "STATUS" <- "Idle...." ("STATUS")
  }
  "Ke2000 Out" <- w22
  "PS1 Out" <- w21
  n504 = local write "stop During HD/Cycles"(w7) -> ()
  n505 = local write "stop"(w7) -> ()
  n506 = case shown="True" w19 {
    tunnel: [w1872 w1875] -> w2
    tunnel: w13 -> [w1872 w1874]
    frame False {
    }
    frame True {
      n507 = local write "Online"(FALSE ("Online")) -> ()
      n508 = call "WSVCAP SHL Host TL Close.vi"("error in"=w1874) -> ("error out"=w1875:errorcluster)  [unwired: 14 in]
    }
  }
  "error out" <- w2
  n509 = VISA Write(VISA resource name=w14, write buffer="SOUR:FUNC VOLT;VOLT:MODE FIX;RANG 100;LEV 0.0;:SENS:FUNC \"CURR\";CURR:PROT 60E-3;RANG 100E-3;:OUTP OFF", error in (no error)=w13) -> (VISA resource name out=→"VISA resource name out":refnum<visa-resource-name>, error out=→"error out 2":errorcluster)  [unwired: 1 out]
